vi "main_control_YJtoy.vi"() -> ()   [LabVIEW 2021]
uses:
  Addons/DAQ_Pulse_Gen/DAQ_Control_2.ctl
  Addons/DAQ_Pulse_Gen/DAQ_Control_1.ctl
  Ver_2/Config_File_Paths_v2.ctl
  Ver_2/ZI_Data_v2.ctl
  Addons/DAQ_Pulse_Gen/DAQ_Control_3 .ctl
  <vilib>/Utility/file.llb/Write Delimited Spreadsheet (DBL).vi
  <vilib>/gmath/NumericalOptimization/Nonlinear Curve Fit LM formula string.vi
  <vilib>/Utility/error.llb/Error Cluster From Error Code.vi
  <vilib>/ErrorRing/Error Ring.xnode
  <vilib>/Utility/Data Type/NI_Data Type.lvlib
  <vilib>/Analysis/NI_AALPro.lvlib
  <vilib>/gmath/NI_Gmath.lvlib
panel:
  out "Process name":string
  out "Initial_state_name":string
  out "tomography rotation memory (priv) 2":cluster{"Time":dbl[], dbl[]}[](array[cluster])
  out "MaxTime":dbl
  out "Process Array":cluster{"Timing 0":dbl[]}[](array[cluster])
  out "tomography rotation memory (priv)":cluster{"Time":dbl[], dbl[]}[](array[cluster])
  in  "pulses type (priv)":string[](array[string])=["None", "Y pi/2", "X pi/2"]
  in  "stop":bool
  in  "Tab Control":T1(tab)=enum."Design QPT"
  out "Config folder":string
  out "Chennel names\nare correct (?)":bool
  out "Channel map":map{string, i32}(c390)
  out "Pulses map [us]":map{string, dbl}(c390)
  out "Sampling data":T2={"Sample Numbers"=20000000, "Sample  Frequency (Hz)"=20000000}
  out "Resource Address":T3={"ZI Address"="DEV714", "VISA Keithley"="KEITHLEY"}
  in  "Period number":u32
  in  "Period [us]":dbl
  in  "Name of state (initial_state_)":string
  in  "Name of initial_state":u16(ring) items=["initial_state_01", "initial_state_02", "initial_state_03", "initial_state_04", "initial_state_05", "initial_state_06", "initial_state_07", "initial_state_08", "initial_state_09", "initial_state_10"]
  in  "Run tomography":bool
  in  "Run single FID":bool
  in  "Save for tomography":bool
  in  "Save single sequence":bool
  out "Pulses chart":cluster{dbl[], dbl[]}[](graph)
  in  "Reset sequence":bool
  in  "Channel":u16(ring) items=["LD pump", "LD repump", "LD probe", "pulse X", "pulse Y", "pulse Z", "Keithley ARM", "Keithley TRIG", "Accqusition TRIG", "Nonlinear coil", "None", "Tensor light shift", "pulse ZG"]
  in  "Add pulse advanced":bool
  in  "Physical channels":string[](array[string])
  in  "Add pulse":bool
  in  "Time [us]":dbl
  in  "Z pi/2":bool
  in  "Z pi":bool
  in  "Y pi/2":bool
  in  "Y pi":bool
  in  "X pi/2":bool
  in  "X pi":bool
  in  "Add pumping":bool
  in  "Pumping":T4(ring)
  in  "AOC":bool
  in  "X pi/4":bool
  in  "Save initial state":bool
  in  "Save  process":bool
  in  "Name of process (process_)":string
  in  "Name of process":u16(ring) items=["process_01", "process_02", "process_03", "process_04", "process_05", "process_06", "process_07", "process_08", "process_09", "process_10"]
  in  "Y pi/4":bool
  in  "Z pi/4":bool
  in  "Save multi Sequence":bool
  in  "Run QPT":bool
  in  "initial_state_show":u16(ring) items=["initial_state_01.ini", "initial_state_02.ini", "initial_state_03.ini", "initial_state_04.ini", "initial_state_05.ini", "initial_state_06.ini", "initial_state_07.ini", "initial_state_08.ini", "initial_state_09.ini"]
  in  "Choose init states":bool
  in  "State_update":bool
  out "State_List":string[](array[string]) caption="The Choosen States"
  in  "Delete init states":bool
  in  "Show init state":bool
  in  "Process_update":bool
  in  "Process_show":u16(ring) caption="initial_state_show" items=["process_01.ini", "process_02.ini", "process_03.ini", "process_04.ini", "process_05.ini", "process_06.ini", "process_07.ini", "process_08.ini", "process_09.ini", "process_10.ini"]
  in  "Choose the process":bool
  out "The Choosen Process":string
  out "Pulses chart 2":cluster{dbl[], dbl[]}[](graph)
  out "Pulses chart 3":cluster{dbl[], dbl[]}[](graph)
  in  "Save QPT":bool
  in  "Clear All states":bool
  in  "Multi-FID":bool
  in  "save":bool
  out "Rotation signal 3":cluster{"Time":dbl[], "Array":dbl[]}[](graph)
  out "w":dbl format="%#_3f"
  out "q":dbl format="%#_3f"
  out "g2":dbl format="%#_3f"
  out "g1":dbl format="%#_3f"
  out "C":dbl format="%#_3f"
  out "B":dbl format="%#_3f"
  out "A":dbl format="%#_3f"
  in  "Enum":T5(ring)
  in  "Fit model":bool
  out "Rotation signal":cluster{"Time":dbl[], dbl[]}(graph)
  out "Rotation spectrum":waveform(dbl)[](graph)
  out "Differential signal":cluster{"Time":dbl[], "X":dbl[]}[](graph)
  out "Intensity signal":cluster{"Time":dbl[], dbl[]}(graph)
  out "Polarimeter":dbl(knob) scale=-10.0..10.0
  in  "Run single FID 2":bool
  out "Progress":dbl(slide) scale=0.0..100.0
  in  "Number of repetition":u32=1 min=1 step=1
  in  "Signal in X or Y (?)":bool
  in  "Plot type":u16(ring) items=["None + [ None ]", "None + [ Y pi ]", "None + [ Z(pi/2)+Y(pi) ]", "Y pi/2 + [ None ]", "Y pi/2 + [ Y pi ]", "Y pi/2 + [ Z(pi/2)+Y(pi) ]", "X pi/2 + [ None ]", "X pi/2 + [ Y pi ]", "X pi/2 + [ Z(pi/2)+Y(pi) ]"]
  in  "Save raw data (?)":bool
  in  "Save CYCLOPS data (?)":bool
  out "Rotation signal":cluster{"Time":dbl[], dbl[]}(graph)
  in  "Run tomography 2":bool
  in  "Averaging":u8=1 min=1 step=1
  out "Differential signal":cluster{"Time":dbl[], "X":dbl[]}[](graph)
  out "Intensity signal":cluster{"Time":dbl[], dbl[]}(graph)
  out "Progress":dbl(slide) scale=0.0..100.0
  out "Rotation spectrum":waveform(dbl)[](graph)
  out "Rotation":cluster{"Time":dbl[], dbl[]}(graph)
  in  "Save raw data (?) 2":bool
  in  "Save CYCLOPS data (?) 2":bool
  out "Rotation spectrum 2":waveform(dbl)[](graph)
  out "Rotation signal 2":cluster{"Time":dbl[], dbl[]}(graph)
  out "Differential signal 2":cluster{"Time":dbl[], "X":dbl[]}[](graph)
  out "Intensity signal 2":cluster{"Time":dbl[], dbl[]}(graph)
  out "Single Tomography Progress":dbl(slide) scale=0.0..100.0
  out "Rotation 2":cluster{"Time":dbl[], dbl[]}(graph)
  in  "Averaging 2":u8=1 min=1 step=1
  in  "Run QPT 2":bool
  out "Current_QPT_order":i32
  out "QPT Progress":dbl(slide) scale=0.0..100.0
  # "To change that tab you need to go to block diagram"
  # "Probing will be added during saving"
  # "X"
  # "Y"
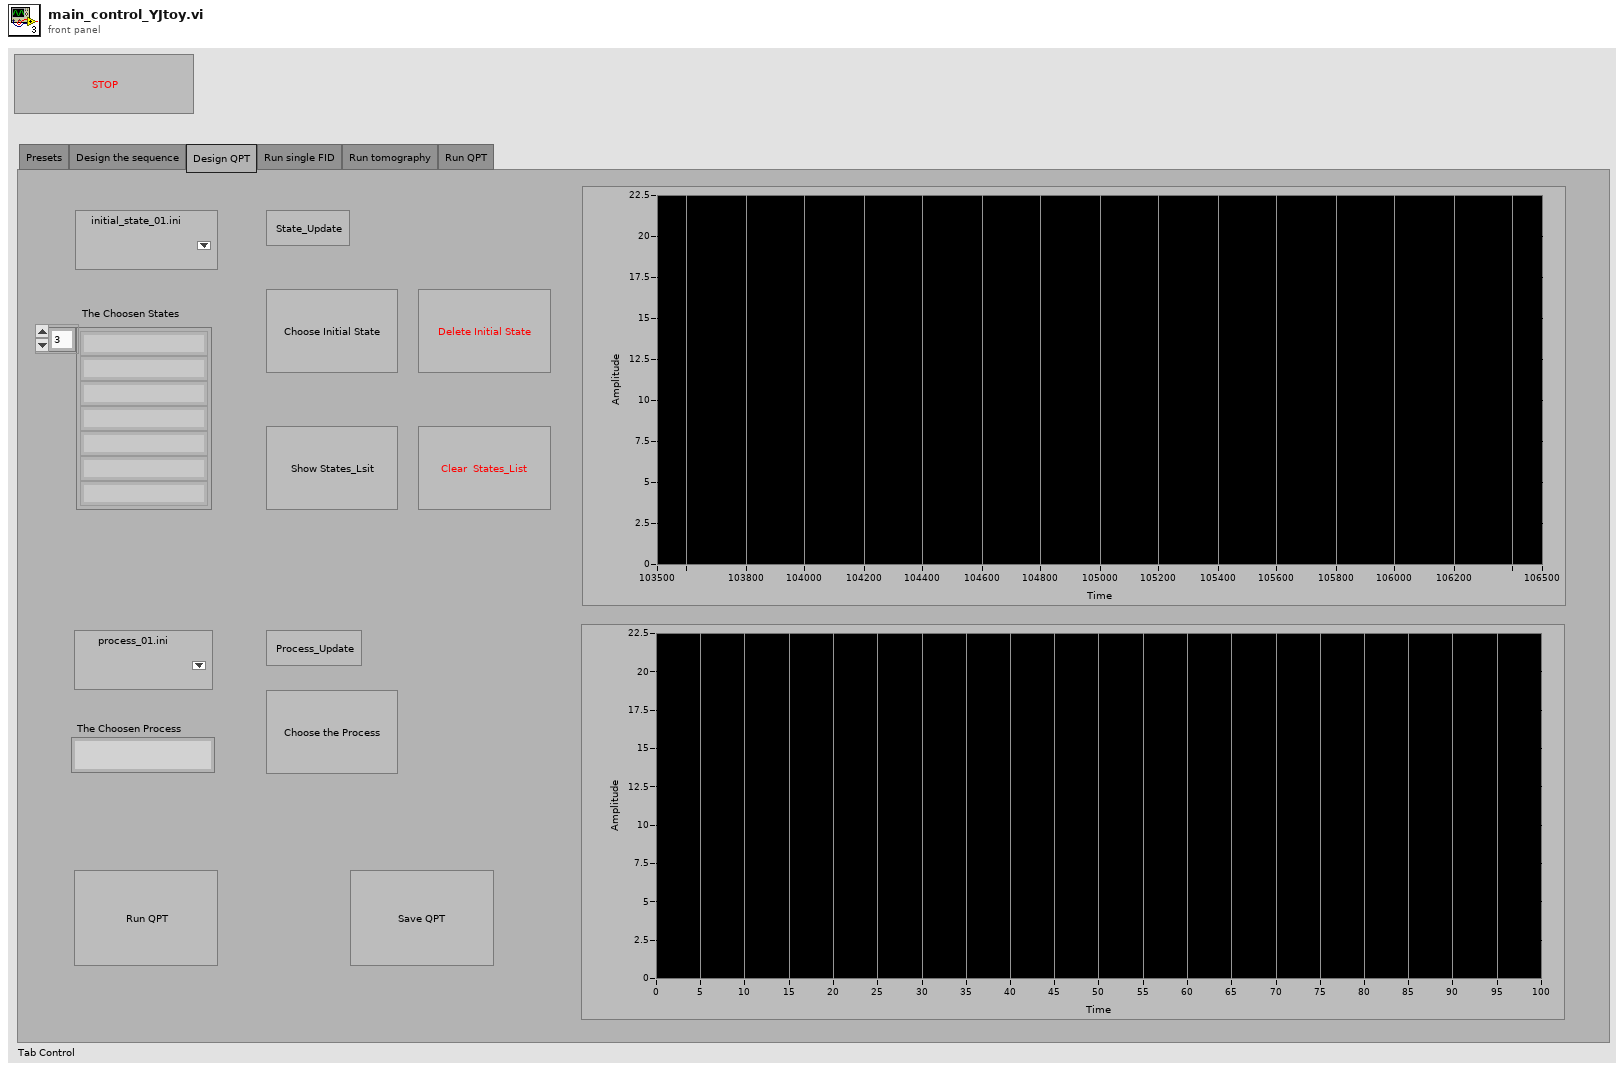
[diagram p1: front panel]
types:
  T1 = enum32{"Presets", "Design the sequence", "Design QPT", "Run single FID", "Run tomography", "Run QPT"}
  T2 = typedef "DAQ_Control_2.ctl" = cluster{"Sample Numbers":u32, "Sample  Frequency (Hz)":u32}
  T3 = cluster{"ZI Address":string, "VISA Keithley":refnum<visa-resource-name>}
  T4 = enum16{"Circular along X", "Linear in Y", "Linear in Z"}
  T5 = enum16{"Full", "A*Sin(w*t+q)*Exp(-g1*t)+C", "B*Exp(-q2*t)+C"}
  T6 = typedef "DAQ_Control_1.ctl" = cluster{"Port 2/line 6":cluster{"Timing 22":dbl[]}, "Port 2/line 5":cluster{"Timing 21":dbl[]}, "Port 2/line 4":cluster{"Timing 20":dbl[]}, "Port 2/line 3":cluster{"Timing 19":dbl[]}, "Port 2/line 2":cluster{"Timing 18":dbl[]}, "Port 2/line 1":cluster{"Timing 17":dbl[]}, "Port 2/line 0":cluster{"Timing 16":dbl[]}, "Port 1/line 7":cluster{"Timing 15":dbl[]}, "Port 1/line 6":cluster{"Timing 14":dbl[]}, "Port 1/line 5":cluster{"Timing 13":dbl[]}, "Port 1/line 4":cluster{"Timing 12":dbl[]}, "Port 1/line 3":cluster{"Timing 11":dbl[]}, "Port 1/line 2":cluster{"Timing 10":dbl[]}, "Port 1/line 1":cluster{"Timing 9":dbl[]}, "Port 1/line 0":cluster{"Timing 8":dbl[]}, "Port 0/line 7":cluster{"Timing 7\n":dbl[]}, "Port 0/line 6":cluster{"Timing 6\n":dbl[]}, "Port 0/line 5":cluster{"Timing 5\n":dbl[]}, "Port 0/line 4":cluster{"Timing 4\n":dbl[]}, "Port 0/line 3":cluster{"Timing 3\n":dbl[]}, "Port 0/line 2":cluster{"Timing 2":dbl[]}, "Port 0/line 1":cluster{"Timing 1\n":dbl[]}, "Port 0/line 0":cluster{"Timing 0":dbl[]}}
  T7 = typedef "Config_File_Paths_v2.ctl" = cluster{"ZI config file (.ini)":string, "Keithley config file (.ini)":string, "DAQ config file (.ini)":string}
  T8 = enum32{"Presets", "Design the sequence", "Design QPT", "Run single FID"}
  T9 = enum8{"Enabled", "Disabled", "Disabled and Grayed Out"}
  T10 = enum32{"Presets", "Design the sequence", "Design QPT", "Run single FID", "Run tomography"}
  T11 = cluster{"model":string, "Parameters":string[], "x":string}
  T12 = typedef "DAQ_Control_3 .ctl" = cluster{"Time Unit":enum16{"NanoSecond", "MicroSecond", "MilliSecond"}}
  T13 = typedef "ZI_Data_v2.ctl" = cluster{"R":dbl[], "Theta":dbl[], "X":dbl[], "Y":dbl[], "AuxIn0":dbl[], "AuxIn1":dbl[], "Frequency":dbl[], "DIO":dbl[], "Time":dbl[]}
  T14 = typedef "Resources_v2.ctl" = cluster{"ZI Handle":T15, "ZI ModHandle":T16, "VISA Keithley":refnum<visa-resource-name>}
  T15 = typedef "Zurich Instruments LabOne.lvlib/ziTypeHandle.ctl" = cluster{"handleValid":bool, "Conn":u64, "Path Prefix":string, "Handle":u64, "Connected":bool, "Clockbase(s)":dbl}
  T16 = typedef "Zurich Instruments LabOne.lvlib/ziTypeModHandle.ctl" = cluster{"handleValid":bool, "Conn":u64, "ModHandle":u64, "moduleID":string, "Path Prefix":string}
  T17 = typedef "Cutted_Data_v2.ctl" = cluster{"X":dbl[], "Y":dbl[], "Time":dbl[]}
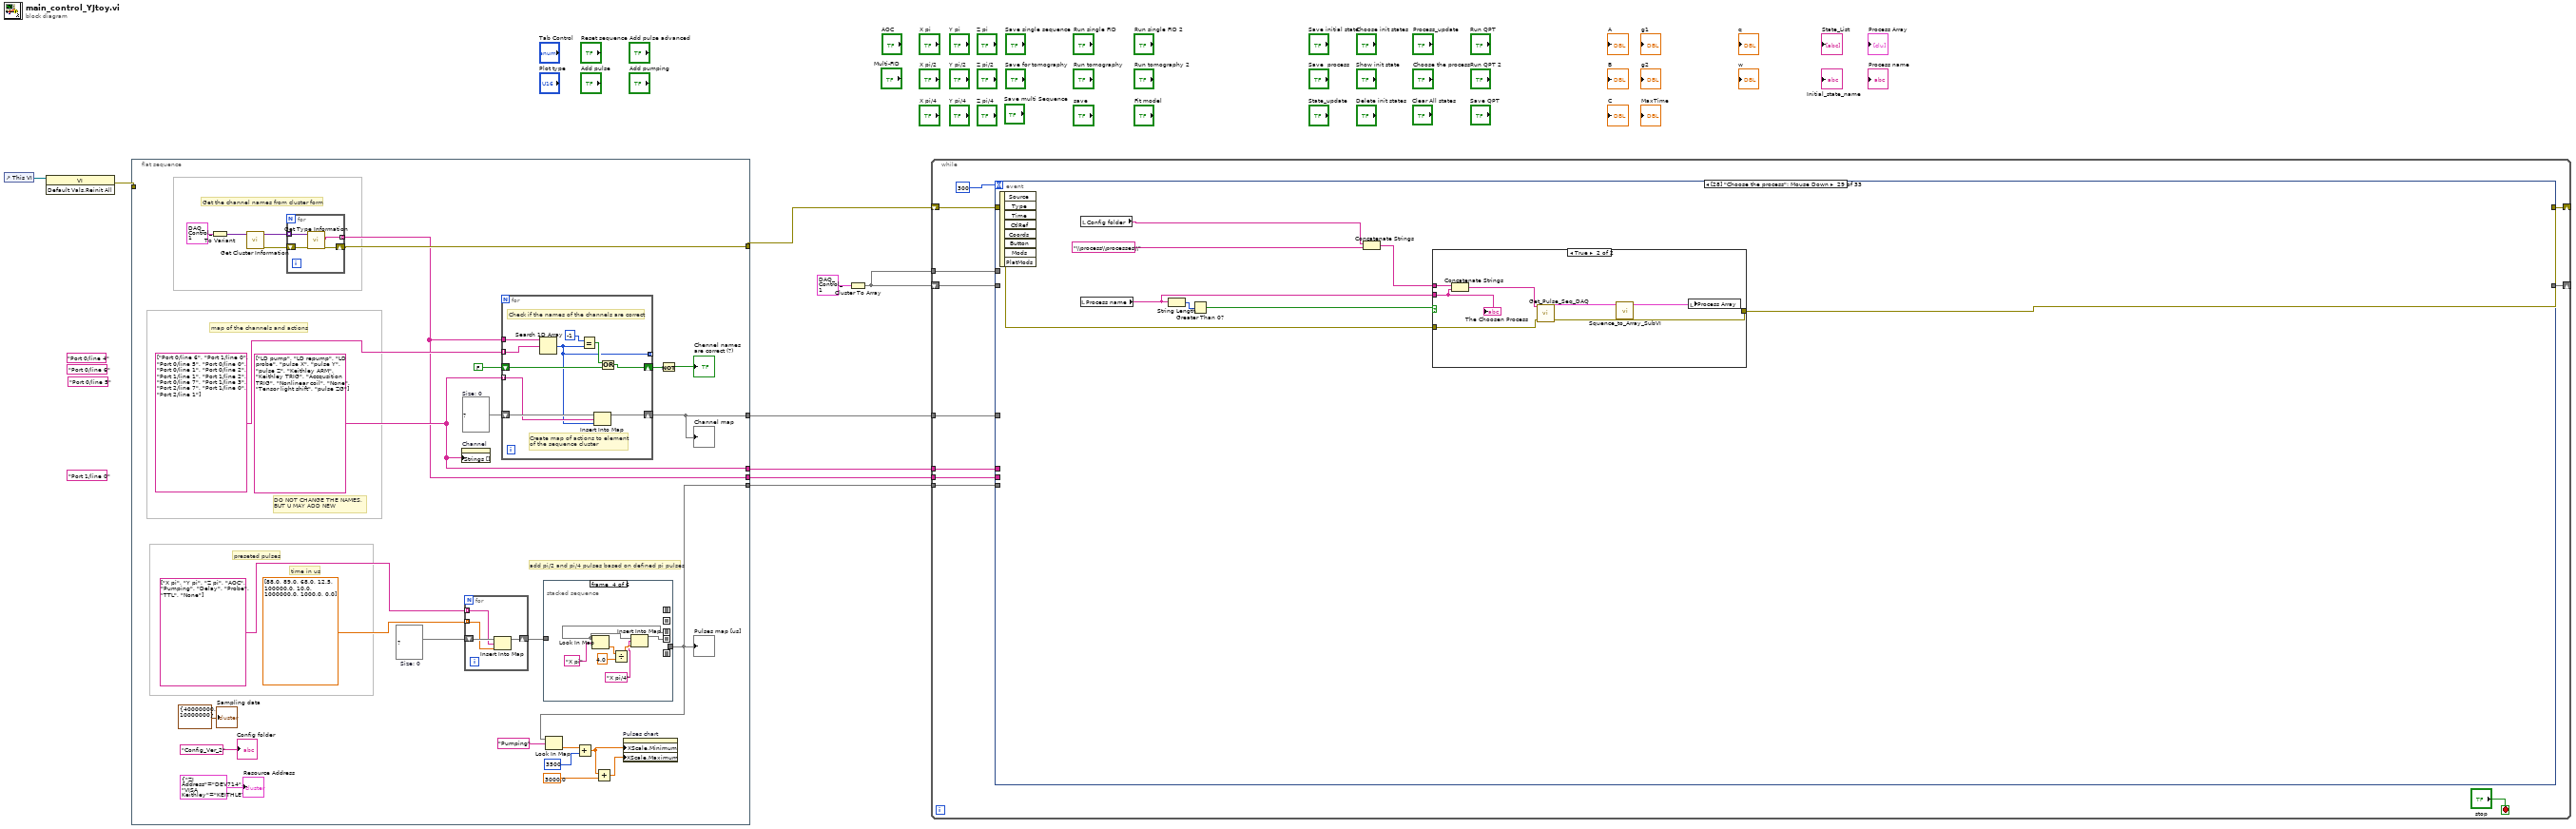
[diagram p0: block diagram]
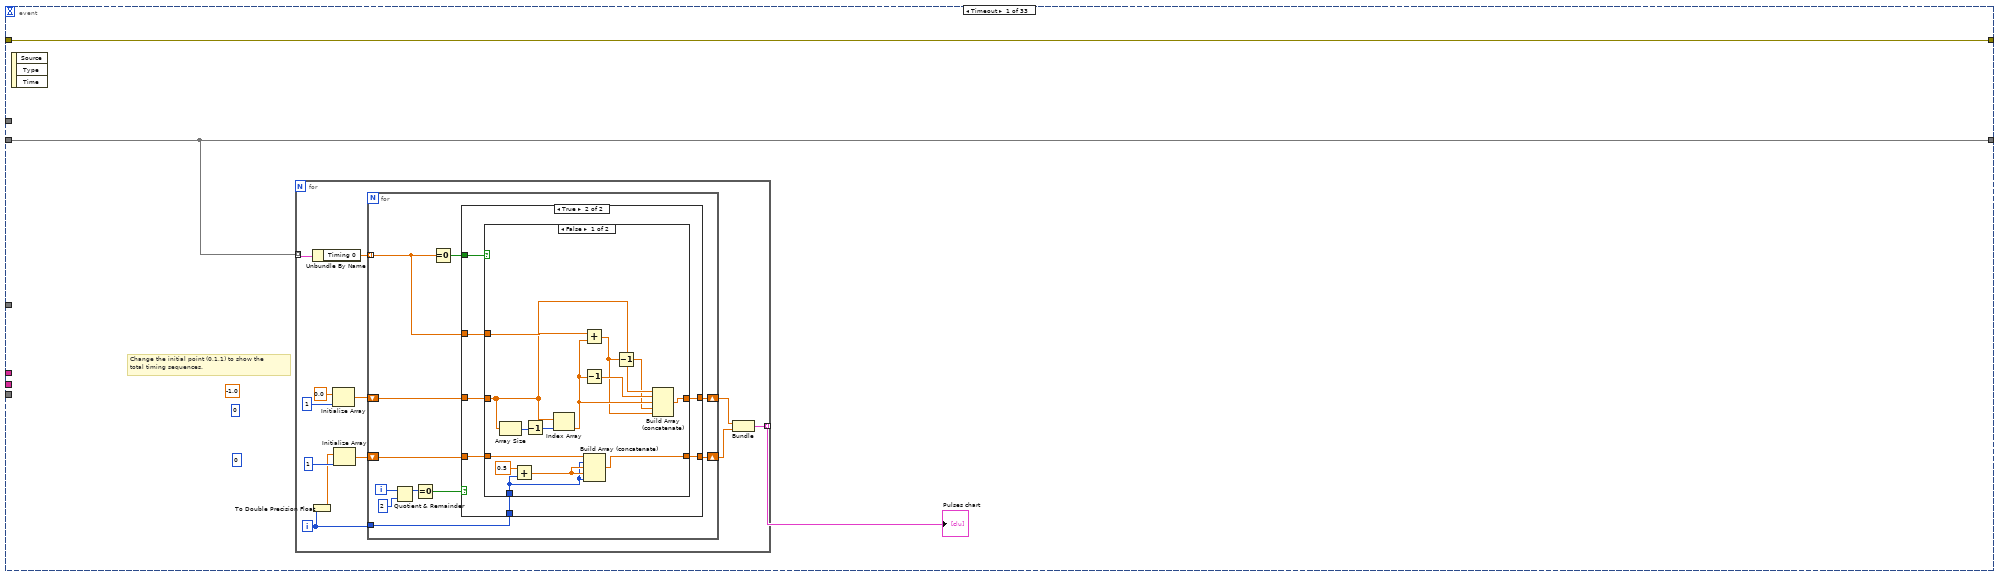
[diagram p2: hidden frame]
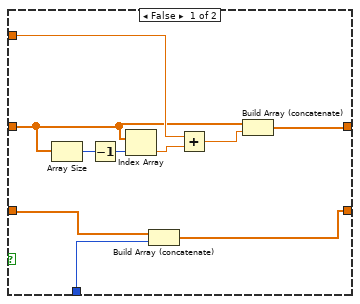
[diagram p3: hidden frame]
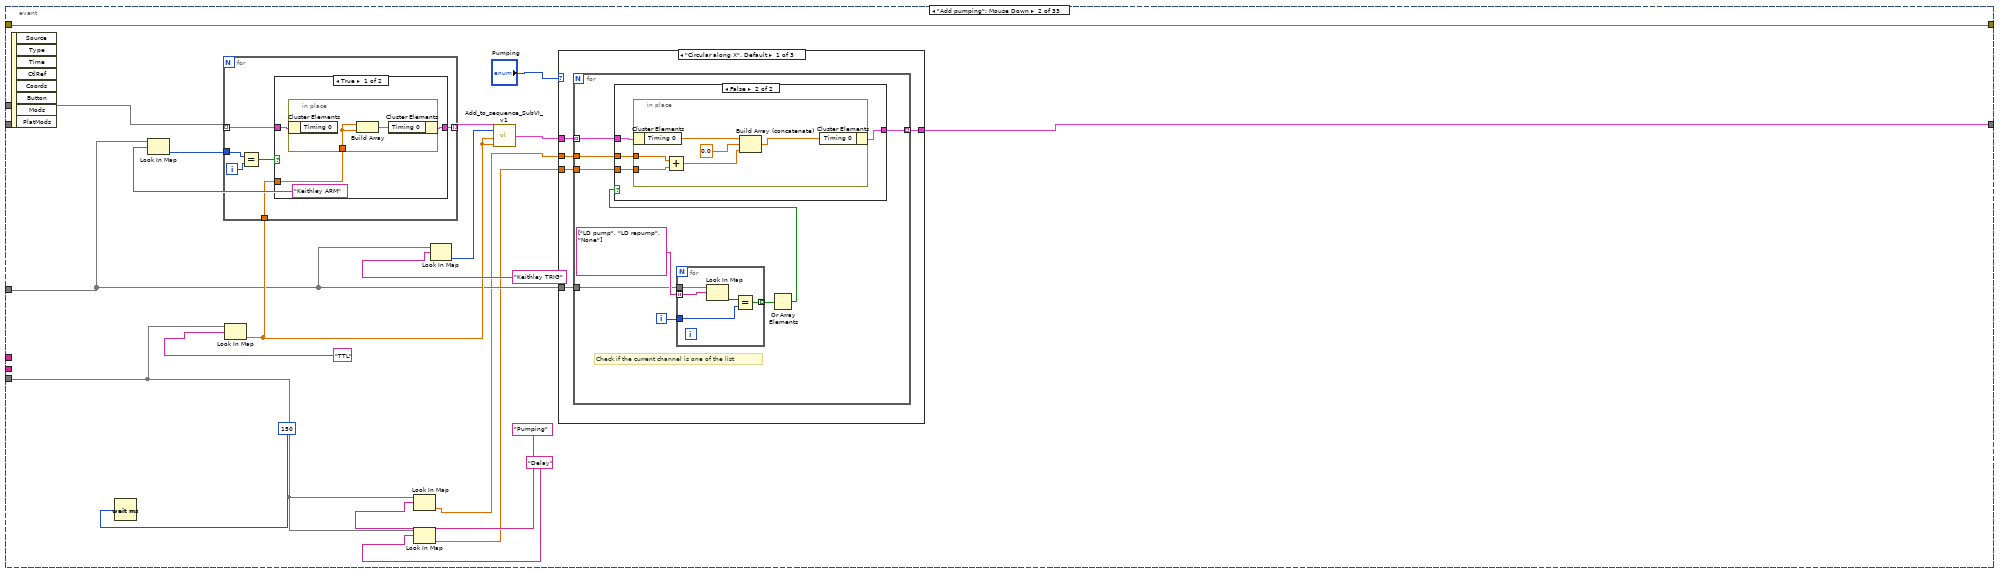
[diagram p5: hidden frame]
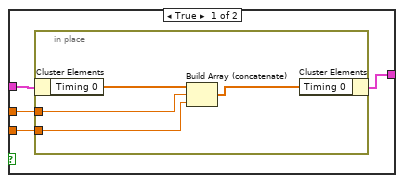
[diagram p6: hidden frame]
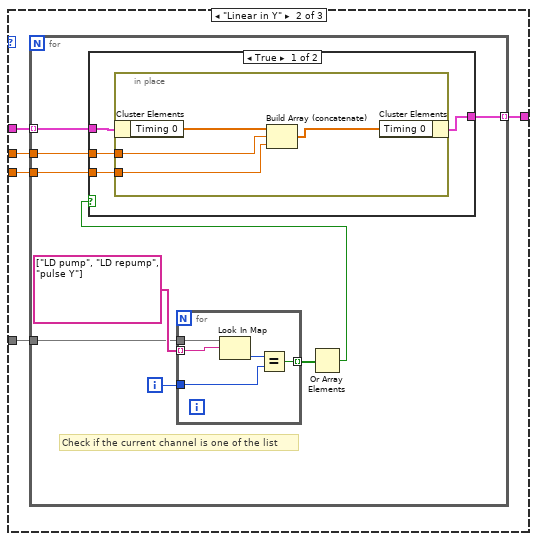
[diagram p7: hidden frame]
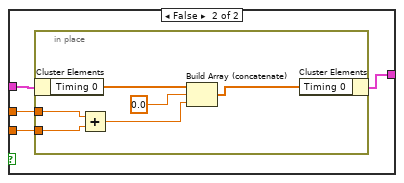
[diagram p8: hidden frame]
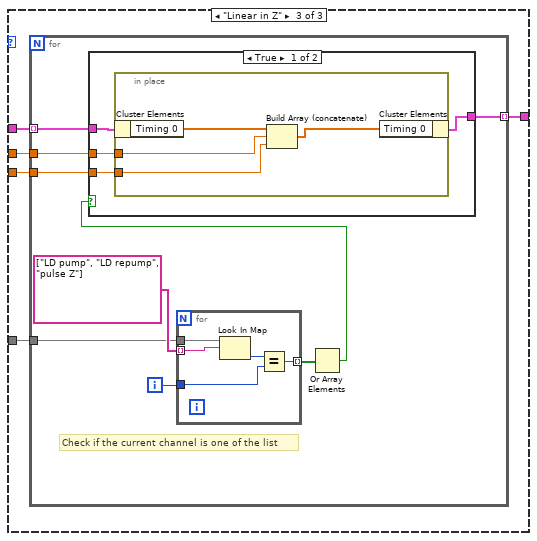
[diagram p9: hidden frame]
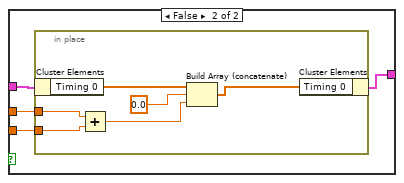
[diagram p10: hidden frame]
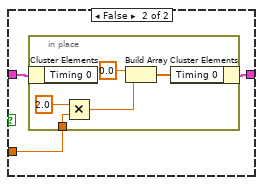
[diagram p11: hidden frame]
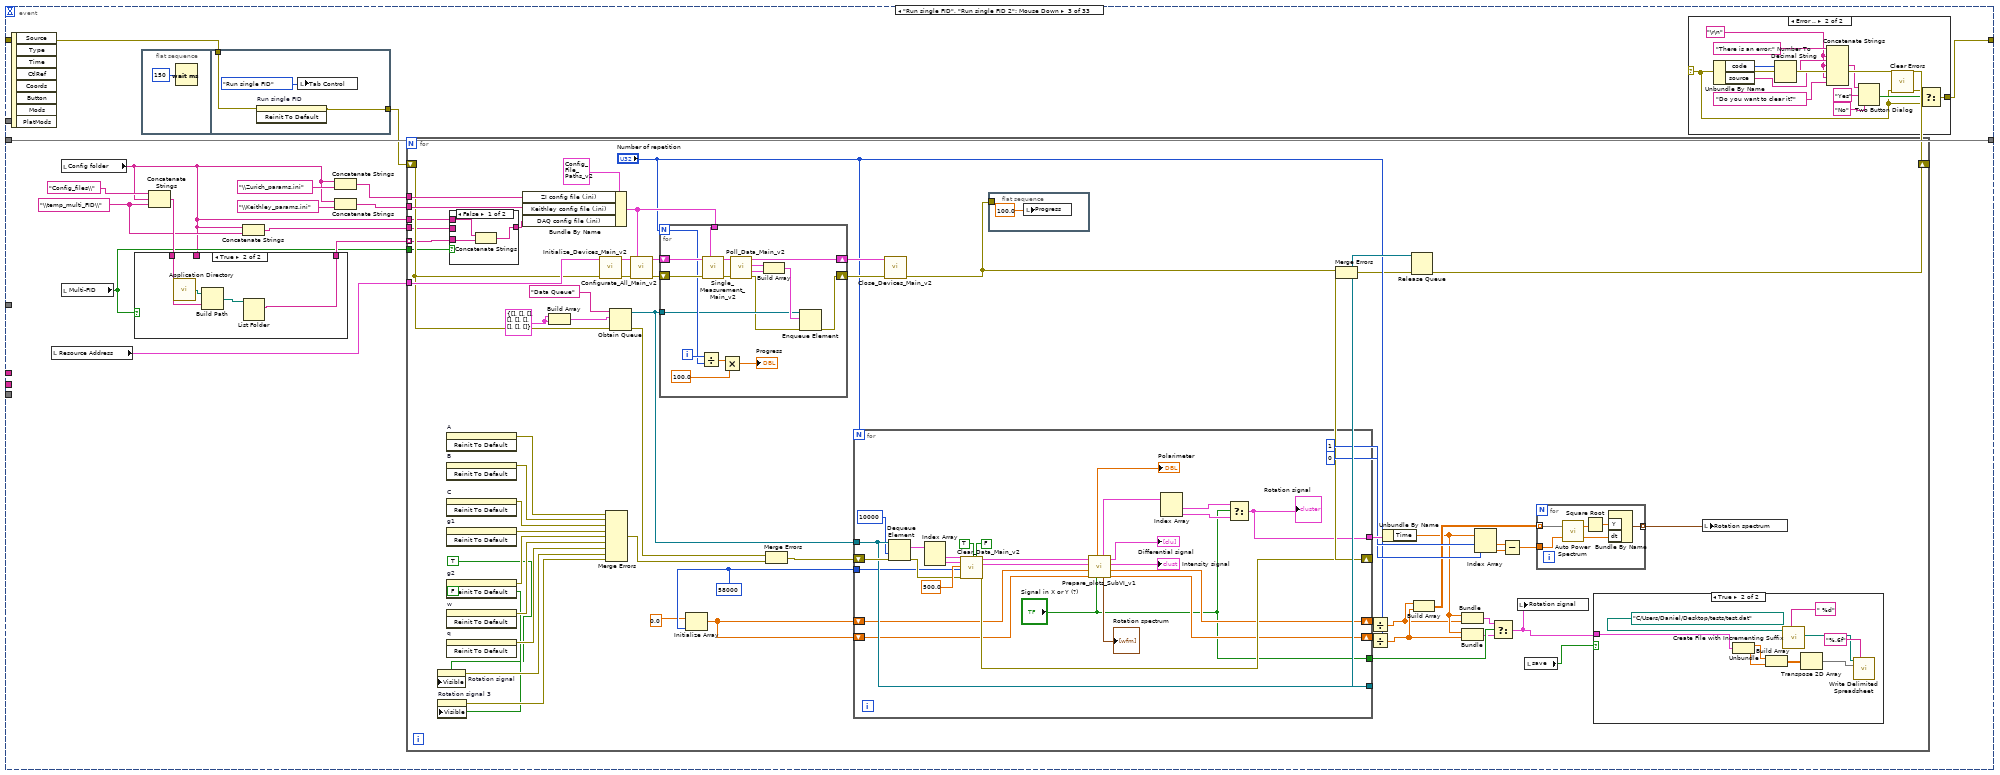
[diagram p12: hidden frame]
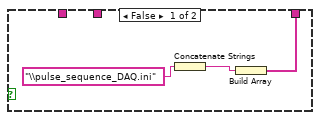
[diagram p13: hidden frame]
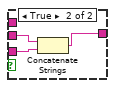
[diagram p14: hidden frame]
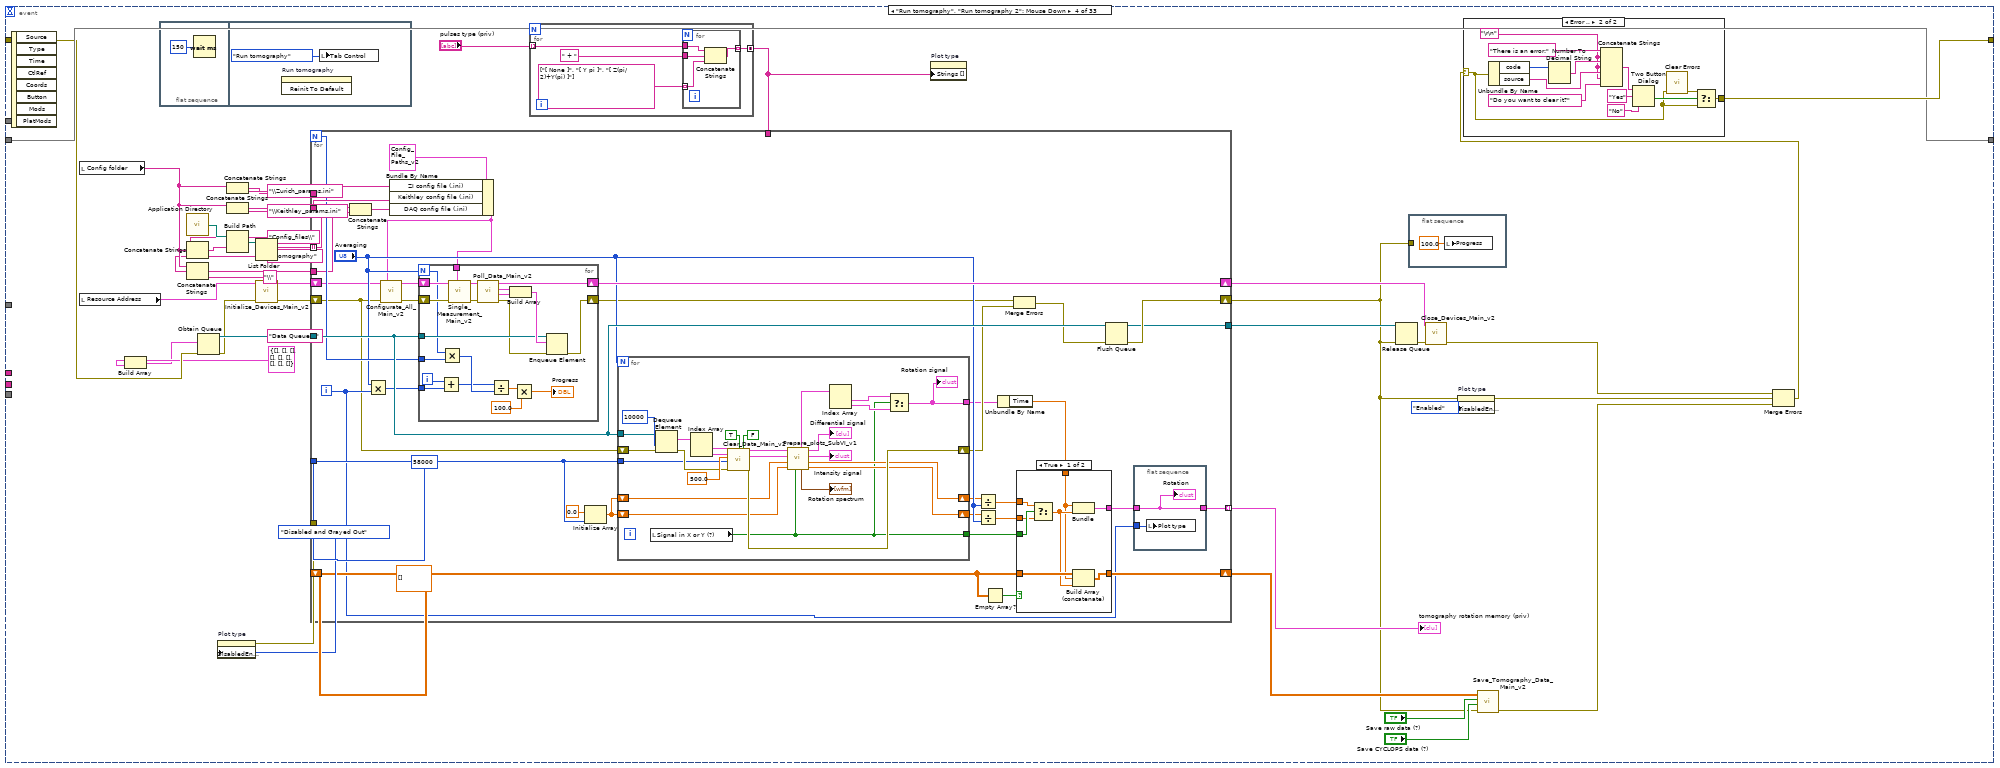
[diagram p17: hidden frame]
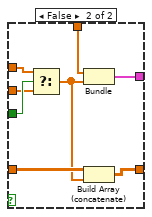
[diagram p18: hidden frame]
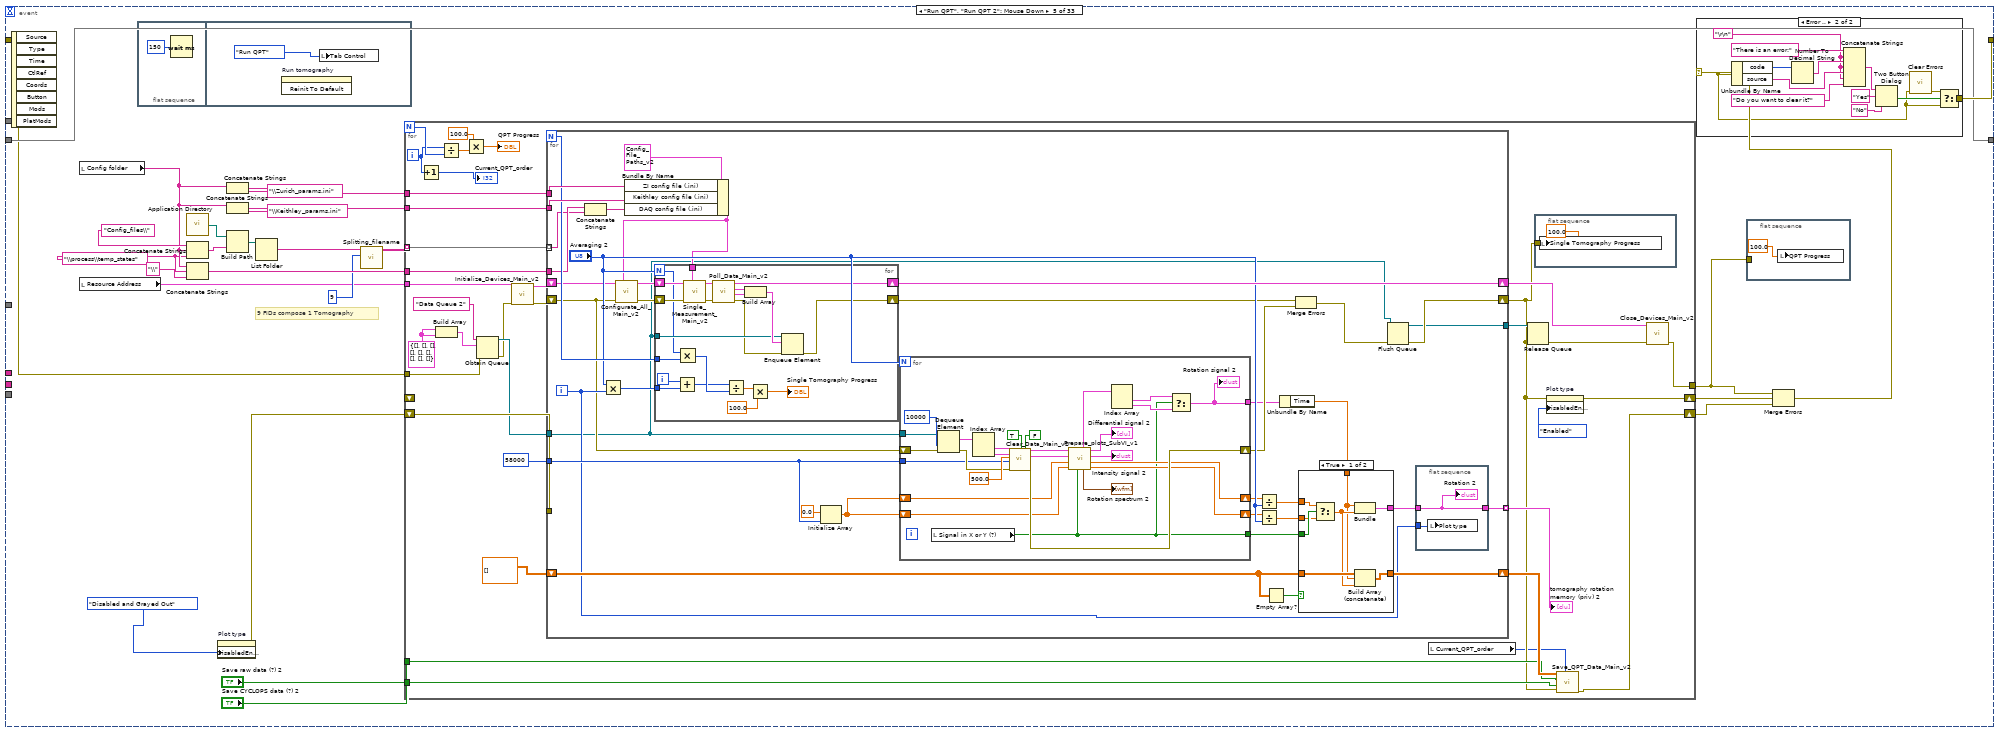
[diagram p20: hidden frame]
diagram:
  (unwired) "Port 0/line 5"
  (unwired) "Port 0/line 4"
  (unwired) "Port 1/line 0"
  (unwired) "Port 0/line 6"
  n1 = control-ref of="This VI"() -> (w2:refnum<vi>)
  n2 = invoke class="VI" method="Default Vals.Reinit All"(reference=w2) -> (error out=w1:errorcluster)  [unwired: 2 in, 2 out]
  n3 = flat-sequence {
    tunnel: [w23] -> w8
    tunnel: [w17] -> w7
    tunnel: [w22] -> w6
    tunnel: [w21] -> w5
    tunnel: [w20] -> w4
    tunnel: w1 -> [_]
    frame #0 {
      w27 = map{string, dbl} {}  # Size: 0
      w29 = map{string, i32} {}  # Size: 0
      w21 = string[] ["LD pump", "LD repump", "LD probe", "pulse X", "pulse Y", "pulse Z", "Keithley ARM", "Keithley TRIG", "Accqusition TRIG", "Nonlinear coil", "None", "Tensor light shift", "pulse ZG"]
      # "DO NOT CHANGE THE NAMES,\nBUT U MAY ADD NEW"
      # "add pi/2 and pi/4 pulses based on defined pi pulses"
      # "preseted pulses"
      # "time in us"
      # "map of the channels and actions"
      # "Get the channel names from cluster form"
      n4 = To Variant(anything=T6 {"Port 2/line 6"={"Timing 22"=[]}, "Port 2/line 5"={"Timing 21"=[]}, "Port 2/line 4"={"Timing 20"=[]}, "Port 2/line 3"={"Timing 19"=[]}, "Port 2/line 2"={"Timing 18"=[]}, "Port 2/line 1"={"Timing 17"=[]}, "Port 2/line 0"={"Timing 16"=[]}, "Port 1/line 7"={"Timing 15"=[]}, "Port 1/line 6"={"Timing 14"=[]}, "Port 1/line 5"={"Timing 13"=[]}, "Port 1/line 4"={"Timing 12"=[]}, "Port 1/line 3"={"Timing 11"=[]}, "Port 1/line 2"={"Timing 10"=[]}, "Port 1/line 1"={"Timing 9"=[]}, "Port 1/line 0"={"Timing 8"=[]}, "Port 0/line 7"={"Timing 7\n"=[]}, "Port 0/line 6"={"Timing 6\n"=[]}, "Port 0/line 5"={"Timing 5\n"=[]}, "Port 0/line 4"={"Timing 4\n"=[]}, "Port 0/line 3"={"Timing 3\n"=[]}, "Port 0/line 2"={"Timing 2"=[]}, "Port 0/line 1"={"Timing 1\n"=[]}, "Port 0/line 0"={"Timing 0"=[]}} ("Sequence")) -> (Variant=w35:variant)
      n5 = call <vilib>:"Get Cluster Information.vi"("variant"=w35) -> ("error out"=w34:errorcluster, "cluster elements"=w33:variant[])  [unwired: 9 in]
      n6 = for {
        tunnel: w33 -> [w96] mode=indexing
        shift-right: [w94] -> w22
        shift-left: w34 -> [w95]
        tunnel: [w93] -> w20 mode=indexing
        n7 = call <vilib>:"Get Type Information.vi"("error in (no error)"=w95, "variant"=w96) -> ("error out"=w94:errorcluster, "name"=w93:string)  [unwired: 5 in, 3 out]
      }
      n8 = property on="Channel" class="Ring (strict)"("Strings []"=w21) -> ()  [unwired: 2 in, 2 out]
      n9 = for {
        shift-right: [w79] -> w24
        shift-left: w27 -> [w82]
        tunnel: string[] ["X pi", "Y pi", "Z pi", "AOC", "Pumping", "Delay", "Probe", "TTL", "None"] -> [w81] mode=indexing
        tunnel: dbl[] [88.0, 89.0, 68.0, 12.5, 100000.0, 10.0, 1000000.0, 1000.0, 0.0] -> [w80] mode=indexing
        n10 = Insert Into Map(map in=w82, key=w81, value=w80) -> (map out=w79:map{string, dbl})  [unwired: 2 out]
      }
      n11 = for {
        tunnel: w20 -> [w92]
        tunnel: string[] ["Port 0/line 6", "Port 1/line 0", "Port 0/line 5", "Port 0/line 0", "Port 0/line 1", "Port 0/line 2", "Port 1/line 1", "Port 1/line 2", "Port 0/line 7", "Port 1/line 3", "Port 2/line 7", "Port 1/line 0", "Port 2/line 1"] -> [w83] mode=indexing
        shift-right: [w88] -> w31
        shift-left: FALSE -> [w89]
        tunnel: [w85] -> _ mode=indexing
        shift-right: [w84] -> w23
        shift-left: w29 -> [w87]
        tunnel: w21 -> [w86] mode=indexing
        # "Create map of actions to element\nof the sequence cluster"
        # "Check if the names of the channels are correct"
        n12 = Search 1D Array(1D array=w92, element=w83) -> (index of element=w85:i32)  [unwired: 1 in]
        n13 = Equal?(x=-1, y=w85) -> (x = y?=w90:bool)
        n14 = Insert Into Map(map in=w87, key=w86, value=w85) -> (map out=w84:map{string, i32})  [unwired: 2 out]
        n15 = Or(x=w90, y=w89) -> (x .or. y?=w88:bool)
      }
      "Channel map" <- w23
      n16 = stacked-sequence {
        seq-local: [w37 _ _ _ _ _] -> [_ w44 _ _ _ _]
        seq-local: [_ w45 _ _ _ _] -> [_ _ w52 _ _ _]
        seq-local: [_ _ w51 _ _ _] -> [_ _ _ w63 _ _]
        seq-local: [_ _ _ w59 _ _] -> [_ _ _ _ w71 _]
        seq-local: [_ _ _ _ w70 _] -> [_ _ _ _ _ w78]
        tunnel: w24 -> [w41 _ _ _ _ _]
        tunnel: [_ _ _ _ _ w77] -> w17
        frame #0 {
          n17 = Look In Map(map=w41, key="X pi") -> (value=w39:dbl)  [unwired: 1 in, 1 out]
          n18 = Divide(x=w39, y=2.0) -> (x/y=w40:dbl)
          n19 = Insert Into Map(map in=w41, key="X pi/2", value=w40) -> (map out=w37:map{string, dbl})  [unwired: 2 out]
        }
        frame #1 {
          n20 = Look In Map(map=w44, key="Y pi") -> (value=w50:dbl)  [unwired: 1 in, 1 out]
          n21 = Divide(x=w50, y=2.0) -> (x/y=w49:dbl)
          n22 = Insert Into Map(map in=w44, key="Y pi/2", value=w49) -> (map out=w45:map{string, dbl})  [unwired: 2 out]
        }
        frame #2 {
          n23 = Look In Map(map=w52, key="Z pi") -> (value=w54:dbl)  [unwired: 1 in, 1 out]
          n24 = Divide(x=w54, y=2.0) -> (x/y=w55:dbl)
          n25 = Insert Into Map(map in=w52, key="Z pi/2", value=w55) -> (map out=w51:map{string, dbl})  [unwired: 2 out]
        }
        frame #3 {
          n26 = Look In Map(map=w63, key="X pi") -> (value=w62:dbl)  [unwired: 1 in, 1 out]
          n27 = Divide(x=w62, y=4.0) -> (x/y=w60:dbl)
          n28 = Insert Into Map(map in=w63, key="X pi/4", value=w60) -> (map out=w59:map{string, dbl})  [unwired: 2 out]
        }
        frame #4 {
          n29 = Look In Map(map=w71, key="Y pi") -> (value=w68:dbl)  [unwired: 1 in, 1 out]
          n30 = Divide(x=w68, y=4.0) -> (x/y=w66:dbl)
          n31 = Insert Into Map(map in=w71, key="Y pi/4", value=w66) -> (map out=w70:map{string, dbl})  [unwired: 2 out]
        }
        frame #5 {
          n32 = Look In Map(map=w78, key="Z pi") -> (value=w75:dbl)  [unwired: 1 in, 1 out]
          n33 = Divide(x=w75, y=4.0) -> (x/y=w73:dbl)
          n34 = Insert Into Map(map in=w78, key="Z pi/4", value=w73) -> (map out=w77:map{string, dbl})  [unwired: 2 out]
        }
      }
      "Pulses map [us]" <- w17
      n35 = Look In Map(map=w17, key="Pumping") -> (value=w19:dbl)  [unwired: 1 in, 1 out]
      n36 = Add(x=w19, y=3500) -> (x+y=w16:dbl)
      n37 = Add(x=w16, y=3000.0) -> (x+y=w14:dbl)
      n38 = property on="Pulses chart" class="XYGraph (strict)"("XScale.Minimum"=w16, "XScale.Maximum"=w14) -> ()  [unwired: 2 in, 2 out]
      n39 = Not(x=w31) -> (.not. x?=→"Chennel names\nare correct (?)":bool)
      "Sampling data" <- T2 {"Sample Numbers"=40000000, "Sample  Frequency (Hz)"=10000000} ("Sampling data")
      "Config folder" <- "Config_Ver_2" ("Filename (ini)")
      "Resource Address" <- T3 {"ZI Address"="DEV714", "VISA Keithley"="KEITHLEY"} ("Resource Address")
    }
  }
  n40 = Cluster To Array(cluster=T6 {"Port 2/line 6"={"Timing 22"=[]}, "Port 2/line 5"={"Timing 21"=[]}, "Port 2/line 4"={"Timing 20"=[]}, "Port 2/line 3"={"Timing 19"=[]}, "Port 2/line 2"={"Timing 18"=[]}, "Port 2/line 1"={"Timing 17"=[]}, "Port 2/line 0"={"Timing 16"=[]}, "Port 1/line 7"={"Timing 15"=[]}, "Port 1/line 6"={"Timing 14"=[]}, "Port 1/line 5"={"Timing 13"=[]}, "Port 1/line 4"={"Timing 12"=[]}, "Port 1/line 3"={"Timing 11"=[]}, "Port 1/line 2"={"Timing 10"=[]}, "Port 1/line 1"={"Timing 9"=[]}, "Port 1/line 0"={"Timing 8"=[]}, "Port 0/line 7"={"Timing 7\n"=[]}, "Port 0/line 6"={"Timing 6\n"=[]}, "Port 0/line 5"={"Timing 5\n"=[]}, "Port 0/line 4"={"Timing 4\n"=[]}, "Port 0/line 3"={"Timing 3\n"=[]}, "Port 0/line 2"={"Timing 2"=[]}, "Port 0/line 1"={"Timing 1\n"=[]}, "Port 0/line 0"={"Timing 0"=[]}} ("Sequence")) -> (array=w3:cluster{"Timing 0":dbl[]}[])
  n41 = while {
    shift-right: [w98] -> _
    shift-left: w3 -> [w107]
    tunnel: w8 -> [w106]
    tunnel: w7 -> [w97]
    shift-right: [w102] -> _
    shift-left: w6 -> [w103]
    tunnel: w5 -> [w101]
    tunnel: w4 -> [w100]
    tunnel: w3 -> [w99]
    stop <- "stop" stop-if-true
    n42 = event shown="[28] \"Choose the process\": Mouse Down" {
      selector: _ -> [_ _ _ _ _ _ _ _ _ _ _ _ _ _ _ _ _ _ _ _ _ _ _ _ _ _ _ _ _ _ _ _ _]
      dyn-events: _ -> [_ _ _ _ _ _ _ _ _ _ _ _ _ _ _ _ _ _ _ _ _ _ _ _ _ _ _ _ _ _ _ _ _]
      timeout: 300 -> [_ _ _ _ _ _ _ _ _ _ _ _ _ _ _ _ _ _ _ _ _ _ _ _ _ _ _ _ _ _ _ _ _]
      tunnel: w107 -> [w110 _ w327 w520 w675 w838 _ w1001 w1006 w1018 w1029 w1041 w1053 w1065 w1077 w1089 w1101 w1117 w1146 w1185 w1266 w1387 w1529 w1576 _ _ _ _ _ _ _ _ _]
      tunnel: w106 -> [_ w172 _ _ _ _ _ w985 w1013 w1025 w1036 w1048 w1060 w1072 w1084 w1096 w1108 w1122 _ w1198 w1268 w1392 _ _ w1640 _ _ _ _ _ _ _ _]
      tunnel: w97 -> [_ w171 _ _ _ _ _ w983 w1007 w1019 w1034 w1042 w1054 w1066 w1078 w1090 w1102 w1118 w1138 w1195 w1267 w1391 _ _ w1639 _ _ _ _ _ _ _ _]
      tunnel: [w110 w169 w327 w520 w675 w838 _ w978 w1005 w1017 w1028 w1040 w1052 w1064 w1076 w1088 w1100 w1116 w1135 w1185 _ w1387 w1529 w1576 _ _ _ _ _ _ _ _ w2013] -> w98
      tunnel: w103 -> [w109 w185 w326 w514 w657 w839 w881 w989 w1009 w1021 _ w1044 w1056 w1068 w1080 w1092 w1104 w1120 w1142 w1180 w1256 w1385 w1530 w1577 w1626 w1737 w1832 w1930 w1949 w1961 w1982 w2010 w2014]
      tunnel: [w109 w185 w324 w524 w678 w839 _ w989 w1009 w1021 _ w1044 w1056 w1068 w1080 w1092 w1104 w1120 w1142 w1179 w1263 w1384 w1531 w1578 w1647 w1736 w1825 w1925 w1943 w1968 w1979 w2009 w2014] -> w102
      tunnel: w101 -> [_ _ _ _ _ _ _ _ _ _ _ _ _ _ _ _ _ w1113 _ _ _ _ _ _ _ _ _ _ _ _ _ _ _]
      tunnel: w100 -> [_ _ _ _ _ _ _ _ _ _ _ _ _ _ _ _ _ _ w1144 _ _ _ _ _ _ _ _ _ _ _ _ _ _]
      tunnel: w99 -> [_ w168 _ _ _ _ _ _ _ _ _ _ _ _ _ _ _ _ _ _ _ _ _ _ _ _ _ _ _ _ _ _ w2013]
      event Timeout {
        (unwired) 0 ("dimension size")
        (unwired) 0 ("dimension size")
        (unwired) -1.0 ("element")
        # "Change the initial point (0,1,1) to show the \ntotal timing sequences."
        n43 = event-data() -> ()  [unwired: 1 in, 3 out]
        n44 = for {
          tunnel: w110 -> [w122] mode=indexing
          tunnel: [w111] -> w108 mode=indexing
          i -> [w114]
          n45 = To Double Precision Float(number=w114) -> (double precision float=w118:dbl)
          n46 = Unbundle By Name(w122) -> ("Timing 0"=w121:dbl[])
          n47 = Initialize Array(0.0 ("element"), 1 ("dimension size")) -> (w115:dbl[])
          n48 = Initialize Array(w118, 1 ("dimension size")) -> (w119:dbl[])
          n49 = for {
            tunnel: w121 -> [w124] mode=indexing
            shift-right: [w126] -> w112
            shift-left: w119 -> [w125]
            shift-right: [w128] -> w113
            shift-left: w115 -> [w127]
            tunnel: w114 -> [w123]
            i -> [w133]
            n50 = Quotient & Remainder(x=w133, y=2) -> (x-y*floor(x/y)=w131:i32)  [unwired: 1 out]
            n51 = Equal To 0?(x=w131) -> (x = 0?=w130:bool)
            n52 = Equal To 0?(x=w124) -> (x = 0?=w129:bool)
            n53 = case shown="True" w130 {
              tunnel: w129 -> [_ w150]
              tunnel: [w134 w149] -> w128
              tunnel: w127 -> [w136 w148]
              tunnel: [w141 w147] -> w126
              tunnel: w125 -> [w142 w146]
              tunnel: w124 -> [w137 w145]
              tunnel: w123 -> [w143 w144]
              frame False {
                n54 = Array Size(array=w136) -> (size(s)=w140:i32)
                n55 = Decrement(x=w140) -> (x-1=w139:i32)
                n56 = Index Array(array=w136, index=w139) -> (element=w138:dbl)
                n57 = Build Array (concatenate)(w142, w143) -> (w141:dbl[])
                n58 = Add(x=w137, y=w138) -> (x+y=w135:dbl)
                n59 = Build Array (concatenate)(w136, w135) -> (w134:dbl[])
              }
              frame True {
                n60 = case shown="False" w150 {
                  tunnel: [w161 w166] -> w149
                  tunnel: w148 -> [w155 w166]
                  tunnel: [w157 w165] -> w147
                  tunnel: w146 -> [w164 w165]
                  tunnel: w145 -> [w162 _]
                  tunnel: w144 -> [w158 _]
                  frame False {
                    n61 = Array Size(array=w155) -> (size(s)=w163:i32)
                    n62 = Add(x=0.5, y=w158) -> (x+y=w159:dbl)
                    n63 = Decrement(x=w163) -> (x-1=w156:i32)
                    n64 = Index Array(array=w155, index=w156) -> (element=w153:dbl)
                    n65 = Add(x=w162, y=w153) -> (x+y=w152:dbl)
                    n66 = Decrement(x=w153) -> (x-1=w154:dbl)
                    n67 = Build Array (concatenate)(w164, w158, w159, w159, w158) -> (w157:dbl[])
                    n68 = Decrement(x=w152) -> (x-1=w151:dbl)
                    n69 = Build Array (concatenate)(w155, w154, w153, w151, w152) -> (w161:dbl[])
                  }
                  frame True {
                  }
                }
              }
            }
          }
          n70 = Bundle(w113, w112) -> (w111:cluster{dbl[], dbl[]})  [unwired: 1 in]
        }
        "Pulses chart" <- w108
      }
      event "Add pumping": Mouse Down {
        n71 = event-data() -> ()  [unwired: 1 in, 8 out]
        n72 = Wait (ms)(milliseconds to wait=u32 150) -> ()  [unwired: 1 out]
        n73 = Look In Map(map=w172, key="Keithley ARM") -> (value=w182:i32)  [unwired: 1 in, 1 out]
        n74 = Look In Map(map=w171, key="TTL") -> (value=w177:dbl)  [unwired: 1 in, 1 out]
        n75 = for {
          tunnel: w168 -> [w299] mode=indexing
          tunnel: w182 -> [w301]
          tunnel: w177 -> [w298]
          tunnel: [w297] -> w180 mode=indexing
          i -> [w302]
          n76 = Equal?(x=w301, y=w302) -> (x = y?=w300:bool)
          n77 = case shown="True" w300 {
            tunnel: w299 -> [w305 w310]
            tunnel: w298 -> [w304 w309]
            tunnel: [w303 w308] -> w297
            frame True {
              n78 = in-place {
                in-place-border: w304 -> [w307]
                n79 = in-place-cluster #1(w305) -> ()  [unwired: 1 out]
                n80 = Build Array(w307, w307) -> (w306:dbl[])
                n81 = in-place-cluster #1("Timing 0"=w306) -> (w303:cluster{"Timing 0":dbl[]})
              }
            }
            frame False {
              n82 = in-place {
                in-place-border: w309 -> [w313]
                n83 = in-place-cluster #2(w310) -> ()  [unwired: 1 out]
                n84 = Multiply(x=2.0, y=w313) -> (x*y=w311:dbl)
                n85 = Build Array(0.0 ("element"), w311) -> (w315:dbl[])
                n86 = in-place-cluster #2("Timing 0"=w315) -> (w308:cluster{"Timing 0":dbl[]})
              }
            }
          }
        }
        n87 = Look In Map(map=w171, key="Pumping") -> (value=w167:dbl)  [unwired: 1 in, 1 out]
        n88 = Look In Map(map=w171, key="Delay") -> (value=w170:dbl)  [unwired: 1 in, 1 out]
        n89 = Look In Map(map=w172, key="Keithley TRIG") -> (value=w178:i32)  [unwired: 1 in, 1 out]
        n90 = call "Add_to_sequence_SubVI_v1.vi"("Delay [us]"=w177, "Pulse length [us]"=w177, "Channel number"=w178, "Array sequence in"=w180) -> ("Array sequence out"=w175:cluster{"Timing 0":dbl[]}[])
        n91 = case shown="\"Circular along X\", Default" "Pumping" {
          tunnel: w175 -> [w190 w227 w264]
          tunnel: w172 -> [w189 w226 w263]
          tunnel: w167 -> [w188 w225 w262]
          tunnel: w170 -> [w187 w224 w261]
          tunnel: [w186 w223 w260] -> w169
          frame "Circular along X", Default {
            n92 = for {
              tunnel: w190 -> [w194] mode=indexing
              tunnel: w189 -> [w196]
              tunnel: w188 -> [w193]
              tunnel: w187 -> [w192]
              tunnel: [w191] -> w186 mode=indexing
              i -> [w197]
              # "Check if the current channel is one of the list"
              n93 = for {
                tunnel: w196 -> [w221]
                tunnel: w197 -> [w220]
                tunnel: [w219] -> w199 mode=indexing
                tunnel: string[] ["LD pump", "LD repump", "None"] -> [w218] mode=indexing
                n94 = Look In Map(map=w221, key=w218) -> (value=w222:i32)  [unwired: 1 in, 1 out]
                n95 = Equal?(x=w222, y=w220) -> (x = y?=w219:bool)
              }
              n96 = Or Array Elements(Boolean array=w199) -> (logical OR=w195:bool)
              n97 = case shown="False" w195 {
                tunnel: w194 -> [w203 w211]
                tunnel: w193 -> [w202 w210]
                tunnel: w192 -> [w201 w209]
                tunnel: [w200 w208] -> w191
                frame True {
                  n98 = in-place {
                    in-place-border: w202 -> [w206]
                    in-place-border: w201 -> [w205]
                    n99 = in-place-cluster #3(w203) -> ("Timing 0"=w207:dbl[])
                    n100 = Build Array (concatenate)(w207, w206, w205) -> (w204:dbl[])
                    n101 = in-place-cluster #3("Timing 0"=w204) -> (w200:cluster{"Timing 0":dbl[]})
                  }
                }
                frame False {
                  n102 = in-place {
                    in-place-border: w210 -> [w215]
                    in-place-border: w209 -> [w214]
                    n103 = in-place-cluster #4(w211) -> ("Timing 0"=w217:dbl[])
                    n104 = Add(x=w215, y=w214) -> (x+y=w213:dbl)
                    n105 = Build Array (concatenate)(w217, 0.0 ("element"), w213) -> (w216:dbl[])
                    n106 = in-place-cluster #4("Timing 0"=w216) -> (w208:cluster{"Timing 0":dbl[]})
                  }
                }
              }
            }
          }
          frame "Linear in Y" {
            n107 = for {
              tunnel: w227 -> [w231] mode=indexing
              tunnel: w226 -> [w233]
              tunnel: w225 -> [w230]
              tunnel: w224 -> [w229]
              tunnel: [w228] -> w223 mode=indexing
              i -> [w234]
              # "Check if the current channel is one of the list"
              n108 = for {
                tunnel: w233 -> [w258]
                tunnel: w234 -> [w257]
                tunnel: [w256] -> w236 mode=indexing
                tunnel: string[] ["LD pump", "LD repump", "pulse Y"] -> [w255] mode=indexing
                n109 = Look In Map(map=w258, key=w255) -> (value=w259:i32)  [unwired: 1 in, 1 out]
                n110 = Equal?(x=w259, y=w257) -> (x = y?=w256:bool)
              }
              n111 = Or Array Elements(Boolean array=w236) -> (logical OR=w232:bool)
              n112 = case shown="True" w232 {
                tunnel: w231 -> [w240 w248]
                tunnel: w230 -> [w239 w247]
                tunnel: w229 -> [w238 w246]
                tunnel: [w237 w245] -> w228
                frame True {
                  n113 = in-place {
                    in-place-border: w239 -> [w243]
                    in-place-border: w238 -> [w242]
                    n114 = in-place-cluster #5(w240) -> ("Timing 0"=w244:dbl[])
                    n115 = Build Array (concatenate)(w244, w243, w242) -> (w241:dbl[])
                    n116 = in-place-cluster #5("Timing 0"=w241) -> (w237:cluster{"Timing 0":dbl[]})
                  }
                }
                frame False {
                  n117 = in-place {
                    in-place-border: w247 -> [w252]
                    in-place-border: w246 -> [w251]
                    n118 = in-place-cluster #6(w248) -> ("Timing 0"=w254:dbl[])
                    n119 = Add(x=w252, y=w251) -> (x+y=w250:dbl)
                    n120 = Build Array (concatenate)(w254, 0.0 ("element"), w250) -> (w253:dbl[])
                    n121 = in-place-cluster #6("Timing 0"=w253) -> (w245:cluster{"Timing 0":dbl[]})
                  }
                }
              }
            }
          }
          frame "Linear in Z" {
            n122 = for {
              tunnel: w264 -> [w268] mode=indexing
              tunnel: w263 -> [w270]
              tunnel: w262 -> [w267]
              tunnel: w261 -> [w266]
              tunnel: [w265] -> w260 mode=indexing
              i -> [w271]
              # "Check if the current channel is one of the list"
              n123 = for {
                tunnel: w270 -> [w295]
                tunnel: w271 -> [w294]
                tunnel: [w293] -> w273 mode=indexing
                tunnel: string[] ["LD pump", "LD repump", "pulse Z"] -> [w292] mode=indexing
                n124 = Look In Map(map=w295, key=w292) -> (value=w296:i32)  [unwired: 1 in, 1 out]
                n125 = Equal?(x=w296, y=w294) -> (x = y?=w293:bool)
              }
              n126 = Or Array Elements(Boolean array=w273) -> (logical OR=w269:bool)
              n127 = case shown="True" w269 {
                tunnel: w268 -> [w277 w285]
                tunnel: w267 -> [w276 w284]
                tunnel: w266 -> [w275 w283]
                tunnel: [w274 w282] -> w265
                frame True {
                  n128 = in-place {
                    in-place-border: w276 -> [w280]
                    in-place-border: w275 -> [w279]
                    n129 = in-place-cluster #7(w277) -> ("Timing 0"=w281:dbl[])
                    n130 = Build Array (concatenate)(w281, w280, w279) -> (w278:dbl[])
                    n131 = in-place-cluster #7("Timing 0"=w278) -> (w274:cluster{"Timing 0":dbl[]})
                  }
                }
                frame False {
                  n132 = in-place {
                    in-place-border: w284 -> [w289]
                    in-place-border: w283 -> [w288]
                    n133 = in-place-cluster #8(w285) -> ("Timing 0"=w291:dbl[])
                    n134 = Add(x=w289, y=w288) -> (x+y=w287:dbl)
                    n135 = Build Array (concatenate)(w291, 0.0 ("element"), w287) -> (w290:dbl[])
                    n136 = in-place-cluster #8("Timing 0"=w290) -> (w282:cluster{"Timing 0":dbl[]})
                  }
                }
              }
            }
          }
        }
      }
      event "Run single FID", "Run single FID 2": Mouse Down {
        w319 = "\\temp_multi_FID\\" ("string")
        n137 = event-data() -> ()  [unwired: 1 in, 8 out]
        n138 = local read "Resource Address"() -> (w332:T3)
        n139 = local read "Config folder"() -> (w316:string)
        n140 = local read "Multi-FID"() -> (w317:bool)
        n141 = flat-sequence {
          tunnel: w326 -> [w484]
          tunnel: [w483] -> w325
          frame #0 {
            n142 = Wait (ms)(milliseconds to wait=u32 150) -> ()  [unwired: 1 out]
          }
          frame #1 {
            n143 = invoke on="Run single FID" class="Bool (strict)" method="Reinit To Default"(error in=w484) -> (error out=w483:errorcluster)  [unwired: 2 in, 2 out]
            n144 = local write "Tab Control"(T8."Run single FID" ("Tab Control")) -> ()
          }
        }
        n145 = Concatenate Strings("Config_files\\" ("string"), w316, w319) -> (w320:string)
        n146 = case shown="True" w317 {
          tunnel: w320 -> [_ w337]
          tunnel: [w333 w336] -> w322
          tunnel: w316 -> [_ _]
          frame False {
            n147 = Concatenate Strings("\\pulse_sequence_DAQ.ini" ("string")) -> (w334:string)
            n148 = Build Array(w334) -> (w333:string[])
          }
          frame True {
            n149 = call <vilib>:"Application Directory.vi"() -> ("Application Directory"=w338:path)
            n150 = Build Path(base path=w338, name or relative path=w337) -> (appended path=w339:path)
            n151 = List Folder(path=w339) -> (filenames=w336:string[])  [unwired: 3 in, 3 out]
          }
        }
        n152 = Concatenate Strings(w316, w319) -> (w318:string)
        n153 = Concatenate Strings(w316, "\\Zurich_params.ini" ("string")) -> (w328:string)
        n154 = Concatenate Strings(w316, "\\Keithley_params.ini" ("string")) -> (w329:string)
        n155 = for {
          tunnel: w332 -> [w401]
          tunnel: w329 -> [w397]
          tunnel: w328 -> [w396]
          shift-right: [w359] -> w323
          shift-left: w325 -> [w389]
          tunnel: w322 -> [w344] mode=indexing
          tunnel: w318 -> [w342]
          tunnel: w317 -> [w341]
          tunnel: w316 -> [w340]
          w363 = T13 {"R"=[], "Theta"=[], "X"=[], "Y"=[], "AuxIn0"=[], "AuxIn1"=[], "Frequency"=[], "DIO"=[], "Time"=[]} ("ZI Data")
          w386 = u16 58000 ("Fixed Number Of Points")
          n156 = property on="Rotation signal" class="XYGraph (strict)"("Visible"=TRUE) -> (error out=w355:errorcluster)  [unwired: 2 in, 1 out]
          n157 = property on="Rotation signal 3" class="XYGraph (strict)"("Visible"=FALSE) -> (error out=w356:errorcluster)  [unwired: 2 in, 1 out]
          n158 = invoke on="A" class="DigNum (strict)" method="Reinit To Default"() -> (error out=w351:errorcluster)  [unwired: 3 in, 2 out]
          n159 = invoke on="B" class="DigNum (strict)" method="Reinit To Default"() -> (error out=w350:errorcluster)  [unwired: 3 in, 2 out]
          n160 = invoke on="C" class="DigNum (strict)" method="Reinit To Default"() -> (error out=w349:errorcluster)  [unwired: 3 in, 2 out]
          n161 = invoke on="g1" class="DigNum (strict)" method="Reinit To Default"() -> (error out=w348:errorcluster)  [unwired: 3 in, 2 out]
          n162 = invoke on="g2" class="DigNum (strict)" method="Reinit To Default"() -> (error out=w352:errorcluster)  [unwired: 3 in, 2 out]
          n163 = invoke on="w" class="DigNum (strict)" method="Reinit To Default"() -> (error out=w353:errorcluster)  [unwired: 3 in, 2 out]
          n164 = invoke on="q" class="DigNum (strict)" method="Reinit To Default"() -> (error out=w354:errorcluster)  [unwired: 3 in, 2 out]
          n165 = case shown="False" w341 {
            tunnel: w344 -> [w404 w407]
            tunnel: [w402 w406] -> w343
            tunnel: w342 -> [_ w405]
            tunnel: w340 -> [w403 _]
            frame False {
              n166 = Concatenate Strings(w403, w404) -> (w402:string)
            }
            frame True {
              n167 = Concatenate Strings(w405, w407) -> (w406:string)
            }
          }
          n168 = Bundle By Name(cluster=T7 {"ZI config file (.ini)"="Config_Ver_2\\Zurich_params.ini", "Keithley config file (.ini)"="Config_Ver_2\\Keithley_params.ini", "DAQ config file (.ini)"="Config_Ver_2\\pulse_sequence_DAQ.ini"} ("Config files paths"), "ZI config file (.ini)"=w396, "Keithley config file (.ini)"=w397, "DAQ config file (.ini)"=w343) -> (w393:T7)
          n169 = Build Array(w363, w363) -> (w362:T13[])
          n170 = call "Initialize_Devices_Main_v2.vi"("error in"=w389, "Resource Address"=w401) -> ("error out"=w399:errorcluster, "Resources"=w400:T14)  [unwired: 8 in]
          n171 = Merge Errors(w351, w350, w349, w348, w352, w353, w354, w355, w356) -> (w345:errorcluster)
          n172 = Obtain Queue(name (unnamed)="Data Queue", element data type=w362, error in (no error)=w389) -> (queue out=w388:refnum<queue>, error out=w365:errorcluster)  [unwired: 2 in, 1 out]
          n173 = call "Configurate_All_Main_v2.vi"("Resources in"=w400, "Config files paths"=w393, "error in"=w399) -> ("Resources out"=w395:T14, "error out"=w394:errorcluster)  [unwired: 6 in, 5 out]
          n174 = for {
            N: "Number of repetition" -> [w460]
            tunnel: w393 -> [w465]
            shift-right: [w464] -> w392
            shift-left: w395 -> [w467]
            shift-right: [w452] -> w391
            shift-left: w394 -> [w466]
            tunnel: w388 -> [w455]
            i -> [w461]
            n175 = Divide(x=w461, y=w460) -> (x/y=w458:dbl)
            n176 = call "Single_Measurement_Main_v2.vi"("Config files paths"=w465, "error in"=w466, "Resources in"=w467) -> ("error out"=w462:errorcluster, "Resources out"=w463:T14)  [unwired: 6 in, 1 out]
            n177 = Multiply(x=w458, y=100.0) -> (x*y=→"Progress":dbl)
            n178 = call "Poll_Data_Main_v2.vi"("error in"=w462, "Resources in"=w463) -> ("error out"=w453:errorcluster, "ZI Data 3"=w454:T13, "ZI Data 0"=w451:T13, "Resources out"=w464:T14)  [unwired: 6 in]
            n179 = Build Array(w451, w454) -> (w456:T13[])
            n180 = Enqueue Element(queue=w455, element=w456, error in (no error)=w453) -> (error out=w452:errorcluster)  [unwired: 1 in, 2 out]
          }
          n181 = Initialize Array(0.0 ("element"), w386) -> (w384:dbl[])
          n182 = Merge Errors(w365, w345) -> (w364:errorcluster)
          n183 = for {
            N: "Number of repetition" -> [_]
            tunnel: w388 -> [w444]
            shift-right: [w441] -> w361
            shift-left: w364 -> [w446]
            tunnel: [w444] -> w387
            shift-right: [w434] -> w369
            shift-left: w384 -> [w437]
            tunnel: w386 -> [w440]
            shift-right: [w435] -> w370
            shift-left: w384 -> [w436]
            tunnel: [w423] -> w383
            tunnel: ["Signal in X or Y (?)"] -> w382
            n184 = Dequeue Element(queue=w444, timeout in ms (-1)=10000, error in (no error)=w446) -> (element=w445:T13[], error out=w442:errorcluster)  [unwired: 2 out]
            n185 = Index Array(array=w445) -> (element #1=w425:T13, element #2=w443:T13)  [unwired: 2 in]
            n186 = call "Clear_Data_Main_v2.vi"("ZI Data 0"=w425, "ZI Data 3"=w443, "Time Of Collected Data (ms)"=500.0, 3:"Fixed Number Of Points"=w440, "error in"=w442, 10:"Fixed Number Of Points"=TRUE ("Fixed Number Of Points"), "Check Phase Mismatch"=FALSE) -> ("Cutted Data 0"=w439:T17, "Cutted Data 3"=w438:T17, "error out"=w441:errorcluster)  [unwired: 7 in, 3 out]
            n187 = call "Prepare_plots_SubVI_v1.vi"("Signal in X or Y (?)"="Signal in X or Y (?)", "Y rot avg in"=w436, "X rot avg in"=w437, "Cutted Data 3"=w438, "Cutted Data 0"=w439) -> ("Y rot avg out"=w435:dbl[], "X rot avg out"=w434:dbl[], "Monitor"=→"Intensity signal":cluster{"Time":dbl[], dbl[]}, "RF out"=→"Differential signal":cluster{"Time":dbl[], "Y":dbl[]}[], "Rotation spectrum"=→"Rotation spectrum":waveform(dbl)[], "Rotation"=w430:cluster{"Time":dbl[], dbl[]}[], "Polarimeter"=→"Polarimeter":dbl)
            n188 = Index Array(array=w430) -> (element #1=w429:cluster{"Time":dbl[], dbl[]}, element #2=w428:cluster{"Time":dbl[], dbl[]})  [unwired: 2 in]
            n189 = Select(t=w429, s="Signal in X or Y (?)", f=w428) -> (s? t:f=w423:cluster{"Time":dbl[], dbl[]})
            "Rotation signal" <- w423
          }
          n190 = call "Close_Devices_Main_v2.vi"("error in"=w391, "Resources"=w392) -> ("error out"=w371:errorcluster)  [unwired: 9 in]
          n191 = flat-sequence {
            tunnel: w371 -> [_]
            frame #0 {
              n192 = local write "Progress"(100.0 ("Progress")) -> ()
            }
          }
          n193 = Merge Errors(w371, w361) -> (w360:errorcluster)
          n194 = Divide(x=w369, y="Number of repetition") -> (x/y=w367:dbl[])
          n195 = Divide(x=w370, y="Number of repetition") -> (x/y=w368:dbl[])
          n196 = Unbundle By Name(w383) -> ("Time"=w374:dbl[])
          n197 = Release Queue(queue=w387, error in (no error)=w360) -> (error out=w359:errorcluster)  [unwired: 1 in, 2 out]
          n198 = Build Array(w367, w368) -> (w375:dbl[][])
          n199 = Bundle("Time"=w374, w367) -> (w380:cluster{"Time":dbl[], dbl[]})  [unwired: 1 in]
          n200 = Bundle("Time"=w374, w368) -> (w381:cluster{"Time":dbl[], dbl[]})  [unwired: 1 in]
          n201 = Index Array(array=w374, index #1=1 ("index"), index #2=0 ("index")) -> (element #1=w378:dbl, element #2=w379:dbl)
          n202 = Select(t=w380, s=w382, f=w381) -> (s? t:f=w357:cluster{"Time":dbl[], dbl[]})
          n203 = Subtract(x=w378, y=w379) -> (x-y=w373:dbl)
          n204 = local write "Rotation signal"(w357) -> ()
          n205 = local read "save"() -> (w358:bool)
          n206 = for {
            tunnel: w375 -> [w422] mode=indexing
            tunnel: [w420] -> w372 mode=indexing
            tunnel: w373 -> [w417]
            n207 = call <vilib>:"Auto Power Spectrum.vi"("dt"=w417, "Signal (V)"=w422) -> ("df"=w421:dbl, "Power Spectrum (V^2 rms)"=w419:dbl[])
            n208 = Square Root(x=w419) -> (sqrt(x)=w418:dbl[])
            n209 = Bundle By Name("Y"=w418, "dt"=w421) -> (w420:waveform(dbl))  [unwired: 1 in]
          }
          n210 = case shown="True" w358 {
            tunnel: w357 -> [_ w416]
            frame False {
            }
            frame True {
              n211 = Unbundle(w416) -> ("Time"=w415:dbl[], w414:dbl[])
              n212 = Build Array(w415, w414) -> (w413:dbl[][])
              n213 = call <vilib>:"Create File with Incrementing Suffix.vi"("format string (\" (%d)\")"=" %d" ("format string (\" (%d)\")"), "file path"=path "C:/Users/Daniel/Desktop/tests/test.dat") -> ("actual path"=w410:path)  [unwired: 7 in, 2 out]
              n214 = Transpose 2D Array(2D array=w413) -> (transposed array=w412:dbl[][])
              n215 = call-poly <vilib>:"Write Delimited Spreadsheet.vi"("file path (dialog if empty)"=w410, "format (%.3f)"="%.6f", "2D data"=w412) -> ()  [unwired: 11 in, 2 out]
            }
          }
          n216 = local write "Rotation spectrum"(w372) -> ()
        }
        n217 = case shown="Error .." w323 {
          selector: w323 -> [w468 w469]
          tunnel: [w468 w472] -> w324
          frame No Error {
          }
          frame Error {
            w477 = "\r\n"
            n218 = Unbundle By Name(w469) -> ("code"=w480:i32, "source"=w478:string)
            n219 = Number To Decimal String(number=w480) -> (decimal integer string=w479:string)  [unwired: 1 in]
            n220 = Concatenate Strings("There is an error:" ("string"), w477, w479, w477, w478, w477, "Do you want to clear it?" ("string")) -> (w473:string)
            n221 = Two Button Dialog(message=w473, 1:"No" ("F button name (\"Cancel\")"), 2:"Yes" ("T button name (\"OK\")")) -> (T button?=w471:bool)
            n222 = call <vilib>:"Clear Errors.vi"("error in (no error)"=w469) -> ("error out"=w470:errorcluster)  [unwired: 5 in, 1 out]
            n223 = Select(t=w470, s=w471, f=w469) -> (s? t:f=w472:errorcluster)
          }
        }
      }
      event "Run tomography", "Run tomography 2": Mouse Down {
        w494 = T13 {"R"=[], "Theta"=[], "X"=[], "Y"=[], "AuxIn0"=[], "AuxIn1"=[], "Frequency"=[], "DIO"=[], "Time"=[]} ("ZI Data")
        w489 = "\\tomography" ("string")
        n224 = event-data() -> ()  [unwired: 1 in, 8 out]
        n225 = local read "Config folder"() -> (w490:string)
        n226 = local read "Resource Address"() -> (w519:T3)
        n227 = Build Array(w494, w494) -> (w493:T13[])
        n228 = flat-sequence {
          frame #0 {
            n229 = Wait (ms)(milliseconds to wait=u32 150) -> ()  [unwired: 1 out]
          }
          frame #1 {
            n230 = invoke on="Run tomography" class="Bool (strict)" method="Reinit To Default"() -> ()  [unwired: 3 in, 3 out]
            n231 = local write "Tab Control"(T10."Run tomography" ("Tab Control")) -> ()
          }
        }
        n232 = Concatenate Strings("Config_files\\" ("string"), w490, w489) -> (w492:string)
        n233 = Concatenate Strings(w490, w489, "\\" ("string")) -> (w488:string)
        n234 = call <vilib>:"Application Directory.vi"() -> ("Application Directory"=w522:path)
        n235 = Obtain Queue(name (unnamed)="Data Queue 2", element data type=w493, error in (no error)=w514) -> (queue out=w516:refnum<queue>, error out=w513:errorcluster)  [unwired: 2 in, 1 out]
        n236 = property on="Plot type" class="Ring (strict)"("DisabledEnum"=T9."Disabled and Grayed Out" ("Disabled")) -> (error out=w500:errorcluster)  [unwired: 2 in, 1 out]
        n237 = Concatenate Strings(w490, "\\Zurich_params.ini" ("string")) -> (w525:string)
        n238 = Concatenate Strings(w490, "\\Keithley_params.ini" ("string")) -> (w526:string)
        n239 = Build Path(base path=w522, name or relative path=w492) -> (appended path=w523:path)
        n240 = List Folder(path=w523) -> (filenames=w521:string[])  [unwired: 3 in, 3 out]
        n241 = call "Initialize_Devices_Main_v2.vi"("error in"=w513, "Resource Address"=w519) -> ("error out"=w517:errorcluster, "Resources"=w518:T14)  [unwired: 8 in]
        n242 = for {
          tunnel: "pulses type (priv)" -> [w532] mode=indexing
          tunnel: [w530] -> w503 mode=concatenating
          n243 = for {
            tunnel: " + " ("string") -> [w537]
            tunnel: w532 -> [w536]
            tunnel: string[] ["[ None ]", "[ Y pi ]", "[ Z(pi/2)+Y(pi) ]"] -> [w535] mode=indexing
            tunnel: [w534] -> w530 mode=indexing
            n244 = Concatenate Strings(w536, w537, w535) -> (w534:string)
          }
        }
        n245 = for {
          N -> [w566]
          tunnel: w526 -> [w574]
          tunnel: w525 -> [w573]
          tunnel: w521 -> [w538] mode=indexing
          shift-right: [w569] -> w486
          shift-left: w517 -> [w544]
          tunnel: w516 -> [w570]
          shift-right: [w571] -> w512
          shift-left: w518 -> [w543]
          tunnel: u16 58000 ("Fixed Number Of Points") -> [w567]
          tunnel: [w568] -> w510
          shift-right: [w562] -> w507
          shift-left: dbl[][] [] -> [w563]
          tunnel: w503 -> [_]
          tunnel: [w559] -> w502 mode=indexing
          tunnel: w500 -> [_]
          tunnel: w488 -> [w540]
          i -> [w560]
          n246 = Concatenate Strings(w540, w538) -> (w539:string)
          n247 = Multiply(x="Averaging", y=w560) -> (x*y=w565:i32)
          n248 = Bundle By Name(cluster=T7 {"ZI config file (.ini)"="Config_Ver_2\\Zurich_params.ini", "Keithley config file (.ini)"="Config_Ver_2\\Keithley_params.ini", "DAQ config file (.ini)"="Config_Ver_2\\pulse_sequence_DAQ.ini"} ("Config files paths"), "ZI config file (.ini)"=w573, "Keithley config file (.ini)"=w574, "DAQ config file (.ini)"=w539) -> (w541:T7)
          n249 = call "Configurate_All_Main_v2.vi"("Resources in"=w543, "Config files paths"=w541, "error in"=w544) -> ("Resources out"=w542:T14, "error out"=w545:errorcluster)  [unwired: 6 in, 5 out]
          n250 = for {
            N: "Averaging" -> [w623]
            shift-right: [w635] -> w571
            shift-left: w542 -> [w637]
            shift-right: [w626] -> w557
            shift-left: w545 -> [w636]
            tunnel: w570 -> [w628]
            tunnel: w541 -> [w625]
            tunnel: w566 -> [w624]
            tunnel: w565 -> [w620]
            i -> [w621]
            n251 = Add(x=w621, y=w620) -> (x+y=w619:i32)
            n252 = Multiply(x=w623, y=w624) -> (x*y=w622:i32)
            n253 = call "Single_Measurement_Main_v2.vi"("Config files paths"=w625, "error in"=w636, "Resources in"=w637) -> ("error out"=w633:errorcluster, "Resources out"=w634:T14)  [unwired: 6 in, 1 out]
            n254 = call "Poll_Data_Main_v2.vi"("error in"=w633, "Resources in"=w634) -> ("error out"=w627:errorcluster, "ZI Data 3"=w630:T13, "ZI Data 0"=w617:T13, "Resources out"=w635:T14)  [unwired: 6 in]
            n255 = Divide(x=w619, y=w622) -> (x/y=w631:dbl)
            n256 = Build Array(w617, w630) -> (w629:T13[])
            n257 = Multiply(x=w631, y=100.0) -> (x*y=→"Progress":dbl)
            n258 = Enqueue Element(queue=w628, element=w629, error in (no error)=w627) -> (error out=w626:errorcluster)  [unwired: 1 in, 2 out]
          }
          n259 = Initialize Array(0.0 ("element"), w567) -> (w554:dbl[])
          n260 = for {
            N: "Averaging" -> [_]
            shift-right: [w608] -> w558
            shift-left: w544 -> [w613]
            shift-right: [w602] -> w552
            shift-left: w554 -> [w605]
            shift-right: [w603] -> w553
            shift-left: w554 -> [w604]
            tunnel: [w595] -> w548
            tunnel: w570 -> [w594]
            tunnel: w567 -> [w593]
            tunnel: [w592] -> w550
            n261 = local read "Signal in X or Y (?)"() -> (w595:bool)
            n262 = Dequeue Element(queue=w594, timeout in ms (-1)=10000, error in (no error)=w613) -> (element=w612:T13[], error out=w609:errorcluster)  [unwired: 2 out]
            n263 = Index Array(array=w612) -> (element #1=w610:T13, element #2=w611:T13)  [unwired: 2 in]
            n264 = call "Clear_Data_Main_v2.vi"("ZI Data 0"=w610, "ZI Data 3"=w611, "Time Of Collected Data (ms)"=500.0, 3:"Fixed Number Of Points"=w593, "error in"=w609, 10:"Fixed Number Of Points"=TRUE ("Fixed Number Of Points"), "Check Phase Mismatch"=FALSE) -> ("Cutted Data 0"=w607:T17, "Cutted Data 3"=w606:T17, "error out"=w608:errorcluster)  [unwired: 7 in, 3 out]
            n265 = call "Prepare_plots_SubVI_v1.vi"("Signal in X or Y (?)"=w595, "Y rot avg in"=w604, "X rot avg in"=w605, "Cutted Data 3"=w606, "Cutted Data 0"=w607) -> ("Y rot avg out"=w603:dbl[], "X rot avg out"=w602:dbl[], "Monitor"=→"Intensity signal":cluster{"Time":dbl[], dbl[]}, "RF out"=→"Differential signal":cluster{"Time":dbl[], "Y":dbl[]}[], "Rotation spectrum"=→"Rotation spectrum":waveform(dbl)[], "Rotation"=w599:cluster{"Time":dbl[], dbl[]}[])  [unwired: 1 out]
            n266 = Index Array(array=w599) -> (element #1=w598:cluster{"Time":dbl[], dbl[]}, element #2=w597:cluster{"Time":dbl[], dbl[]})  [unwired: 2 in]
            n267 = Select(t=w598, s=w595, f=w597) -> (s? t:f=w592:cluster{"Time":dbl[], dbl[]})
            "Rotation signal" <- w592
          }
          n268 = Divide(x=w552, y="Averaging") -> (x/y=w546:dbl[])
          n269 = Divide(x=w553, y="Averaging") -> (x/y=w547:dbl[])
          n270 = Empty Array?(array=w563) -> (empty?=w551:bool)
          n271 = Unbundle By Name(w550) -> ("Time"=w549:dbl[])
          n272 = Merge Errors(w557, w558) -> (w556:errorcluster)
          n273 = case shown="True" w551 {
            tunnel: w549 -> [w576 w583]
            tunnel: w563 -> [w582 w590]
            tunnel: [w581 w589] -> w562
            tunnel: w548 -> [w580 w588]
            tunnel: w547 -> [w579 w587]
            tunnel: w546 -> [w578 w586]
            tunnel: [w575 w585] -> w561
            frame True {
              n274 = Select(t=w578, s=w580, f=w579) -> (s? t:f=w577:dbl[])
              n275 = Bundle("Time"=w576, w577) -> (w575:cluster{"Time":dbl[], dbl[]})  [unwired: 1 in]
              n276 = Build Array (concatenate)(w582, w576, w577) -> (w581:dbl[][])
            }
            frame False {
              n277 = Select(t=w586, s=w588, f=w587) -> (s? t:f=w584:dbl[])
              n278 = Bundle("Time"=w583, w584) -> (w585:cluster{"Time":dbl[], dbl[]})  [unwired: 1 in]
              n279 = Build Array (concatenate)(w590, w584) -> (w589:dbl[][])
            }
          }
          n280 = Flush Queue(queue=w570, error in (no error)=w556) -> (queue out=w568:refnum<queue>, error out=w569:errorcluster)  [unwired: 1 out]
          n281 = flat-sequence {
            tunnel: w561 -> [w638]
            tunnel: w560 -> [w639]
            tunnel: [w638] -> w559
            frame #0 {
              n282 = local write "Plot type"(w639) -> ()
              "Rotation" <- w638
            }
          }
        }
        "tomography rotation memory (priv)" <- w502
        n283 = property on="Plot type" class="Ring (strict)"("Strings []"=w503) -> ()  [unwired: 2 in, 2 out]
        n284 = Release Queue(queue=w510, error in (no error)=w486) -> (error out=w509:errorcluster)  [unwired: 1 in, 2 out]
        n285 = flat-sequence {
          tunnel: w486 -> [_]
          frame #0 {
            n286 = local write "Progress"(100.0 ("Progress")) -> ()
          }
        }
        n287 = call "Close_Devices_Main_v2.vi"("error in"=w509, "Resources"=w512) -> ("error out"=w498:errorcluster)  [unwired: 9 in]
        n288 = property on="Plot type" class="Ring (strict)"(error in=w486, "DisabledEnum"=T9."Enabled" ("Disabled")) -> (error out=w497:errorcluster)  [unwired: 1 in, 1 out]
        n289 = call "Save_Tomography_Data_Main_v2.vi"("error in"=w486, "Save CYCLOPS data (?)"="Save CYCLOPS data (?)", "Save raw data (?)"="Save raw data (?)", "Data Raw"=w507) -> ("error out"=w496:errorcluster)  [unwired: 6 in, 1 out]
        n290 = Merge Errors(w498, w497, w496) -> (w495:errorcluster)
        n291 = case shown="Error .." w495 {
          selector: w495 -> [w640 w641]
          tunnel: [w640 w644] -> w524
          frame No Error {
          }
          frame Error {
            w649 = "\r\n"
            n292 = Unbundle By Name(w641) -> ("code"=w652:i32, "source"=w650:string)
            n293 = Number To Decimal String(number=w652) -> (decimal integer string=w651:string)  [unwired: 1 in]
            n294 = Concatenate Strings("There is an error:" ("string"), w649, w651, w649, w650, w649, "Do you want to clear it?" ("string")) -> (w645:string)
            n295 = Two Button Dialog(message=w645, 1:"No" ("F button name (\"Cancel\")"), 2:"Yes" ("T button name (\"OK\")")) -> (T button?=w643:bool)
            n296 = call <vilib>:"Clear Errors.vi"("error in (no error)"=w641) -> ("error out"=w642:errorcluster)  [unwired: 5 in, 1 out]
            n297 = Select(t=w642, s=w643, f=w641) -> (s? t:f=w644:errorcluster)
          }
        }
      }
      event "Run QPT", "Run QPT 2": Mouse Down {
        w665 = "\\process\\temp_states" ("string")
        # "9 FIDs compose 1 Tomography"
        n298 = event-data() -> ()  [unwired: 1 in, 8 out]
        n299 = local read "Config folder"() -> (w666:string)
        n300 = local read "Resource Address"() -> (w658:T3)
        n301 = flat-sequence {
          frame #0 {
            n302 = Wait (ms)(milliseconds to wait=u32 150) -> ()  [unwired: 1 out]
          }
          frame #1 {
            n303 = invoke on="Run tomography" class="Bool (strict)" method="Reinit To Default"() -> ()  [unwired: 3 in, 3 out]
            n304 = local write "Tab Control"(T1."Run QPT" ("Tab Control")) -> ()
          }
        }
        n305 = Concatenate Strings("Config_files\\" ("string"), w666, w665) -> (w668:string)
        n306 = Concatenate Strings(w666, w665, "\\" ("string")) -> (w664:string)
        n307 = call <vilib>:"Application Directory.vi"() -> ("Application Directory"=w676:path)
        n308 = property on="Plot type" class="Ring (strict)"("DisabledEnum"=T9."Disabled and Grayed Out" ("Disabled")) -> (error out=w662:errorcluster)  [unwired: 2 in, 1 out]
        n309 = Concatenate Strings(w666, "\\Zurich_params.ini" ("string")) -> (w679:string)
        n310 = Concatenate Strings(w666, "\\Keithley_params.ini" ("string")) -> (w680:string)
        n311 = Build Path(base path=w676, name or relative path=w668) -> (appended path=w677:path)
        n312 = List Folder(path=w677) -> (filenames=w661:string[])  [unwired: 3 in, 3 out]
        n313 = call "Splitting_filename.vi"("Splitting number"=u32 9, "Total filenames"=w661) -> ("Splitted filenames"=w660:string[][])  [unwired: 9 in]
        n314 = for {
          N -> [w707]
          tunnel: w680 -> [w718]
          tunnel: w679 -> [w717]
          tunnel: "Save CYCLOPS data (?) 2" -> [w687]
          tunnel: "Save raw data (?) 2" -> [w688]
          tunnel: w664 -> [w714]
          tunnel: w660 -> [w713] mode=indexing
          shift-right: [w715] -> w671
          shift-left: _ -> [_]
          shift-right: [w685] -> w670
          shift-left: w662 -> [w712]
          tunnel: w658 -> [w703]
          tunnel: w657 -> [w700]
          tunnel: [w692] -> w656
          i -> [w690]
          w697 = T13 {"R"=[], "Theta"=[], "X"=[], "Y"=[], "AuxIn0"=[], "AuxIn1"=[], "Frequency"=[], "DIO"=[], "Time"=[]} ("ZI Data")
          n315 = Increment(x=w690) -> (x+1=→"Current_QPT_order":i32)
          n316 = Build Array(w697, w697) -> (w696:T13[])
          n317 = Divide(x=w690, y=w707) -> (x/y=w706:dbl)
          n318 = Multiply(x=100.0, y=w706) -> (x*y=→"QPT Progress":dbl)
          n319 = Obtain Queue(name (unnamed)="Data Queue 2", element data type=w696, error in (no error)=w700) -> (queue out=w699:refnum<queue>, error out=w698:errorcluster)  [unwired: 2 in, 1 out]
          n320 = call "Initialize_Devices_Main_v2.vi"("error in"=w698, "Resource Address"=w703) -> ("error out"=w702:errorcluster, "Resources"=w701:T14)  [unwired: 8 in]
          n321 = for {
            N -> [w749]
            tunnel: w718 -> [w756]
            tunnel: w717 -> [w755]
            tunnel: w713 -> [w721] mode=indexing
            shift-right: [w752] -> w686
            shift-left: w702 -> [w727]
            shift-right: [w753] -> w693
            shift-left: w701 -> [w726]
            tunnel: u16 58000 ("Fixed Number Of Points") -> [w750]
            tunnel: [w751] -> w711
            shift-right: [w745] -> w689
            shift-left: dbl[][] [] -> [w746]
            tunnel: [w742] -> w708 mode=indexing
            tunnel: w714 -> [w723]
            tunnel: w712 -> [_]
            tunnel: w699 -> [w720]
            i -> [w743]
            n322 = Concatenate Strings(w723, w721) -> (w722:string)
            n323 = Multiply(x="Averaging 2", y=w743) -> (x*y=w748:i32)
            n324 = Bundle By Name(cluster=T7 {"ZI config file (.ini)"="Config_Ver_2\\Zurich_params.ini", "Keithley config file (.ini)"="Config_Ver_2\\Keithley_params.ini", "DAQ config file (.ini)"="Config_Ver_2\\pulse_sequence_DAQ.ini"} ("Config files paths"), "ZI config file (.ini)"=w755, "Keithley config file (.ini)"=w756, "DAQ config file (.ini)"=w722) -> (w724:T7)
            n325 = call "Configurate_All_Main_v2.vi"("Resources in"=w726, "Config files paths"=w724, "error in"=w727) -> ("Resources out"=w725:T14, "error out"=w728:errorcluster)  [unwired: 6 in, 5 out]
            n326 = for {
              N: "Averaging 2" -> [w805]
              shift-right: [w817] -> w753
              shift-left: w725 -> [w819]
              shift-right: [w808] -> w740
              shift-left: w728 -> [w818]
              tunnel: w720 -> [w810]
              tunnel: w724 -> [w807]
              tunnel: w749 -> [w806]
              tunnel: w748 -> [w802]
              i -> [w803]
              n327 = Add(x=w803, y=w802) -> (x+y=w801:i32)
              n328 = Multiply(x=w805, y=w806) -> (x*y=w804:i32)
              n329 = call "Single_Measurement_Main_v2.vi"("Config files paths"=w807, "error in"=w818, "Resources in"=w819) -> ("error out"=w815:errorcluster, "Resources out"=w816:T14)  [unwired: 6 in, 1 out]
              n330 = call "Poll_Data_Main_v2.vi"("error in"=w815, "Resources in"=w816) -> ("error out"=w809:errorcluster, "ZI Data 3"=w812:T13, "ZI Data 0"=w799:T13, "Resources out"=w817:T14)  [unwired: 6 in]
              n331 = Divide(x=w801, y=w804) -> (x/y=w813:dbl)
              n332 = Build Array(w799, w812) -> (w811:T13[])
              n333 = Multiply(x=w813, y=100.0) -> (x*y=→"Single Tomography Progress":dbl)
              n334 = Enqueue Element(queue=w810, element=w811, error in (no error)=w809) -> (error out=w808:errorcluster)  [unwired: 1 in, 2 out]
            }
            n335 = Initialize Array(0.0 ("element"), w750) -> (w737:dbl[])
            n336 = for {
              N: "Averaging 2" -> [_]
              shift-right: [w790] -> w741
              shift-left: w727 -> [w795]
              shift-right: [w784] -> w735
              shift-left: w737 -> [w787]
              shift-right: [w785] -> w736
              shift-left: w737 -> [w786]
              tunnel: [w777] -> w731
              tunnel: w720 -> [w776]
              tunnel: w750 -> [w775]
              tunnel: [w774] -> w733
              n337 = local read "Signal in X or Y (?)"() -> (w777:bool)
              n338 = Dequeue Element(queue=w776, timeout in ms (-1)=10000, error in (no error)=w795) -> (element=w794:T13[], error out=w791:errorcluster)  [unwired: 2 out]
              n339 = Index Array(array=w794) -> (element #1=w792:T13, element #2=w793:T13)  [unwired: 2 in]
              n340 = call "Clear_Data_Main_v2.vi"("ZI Data 0"=w792, "ZI Data 3"=w793, "Time Of Collected Data (ms)"=500.0, 3:"Fixed Number Of Points"=w775, "error in"=w791, 10:"Fixed Number Of Points"=TRUE ("Fixed Number Of Points"), "Check Phase Mismatch"=FALSE) -> ("Cutted Data 0"=w789:T17, "Cutted Data 3"=w788:T17, "error out"=w790:errorcluster)  [unwired: 7 in, 3 out]
              n341 = call "Prepare_plots_SubVI_v1.vi"("Signal in X or Y (?)"=w777, "Y rot avg in"=w786, "X rot avg in"=w787, "Cutted Data 3"=w788, "Cutted Data 0"=w789) -> ("Y rot avg out"=w785:dbl[], "X rot avg out"=w784:dbl[], "Monitor"=→"Intensity signal 2":cluster{"Time":dbl[], dbl[]}, "RF out"=→"Differential signal 2":cluster{"Time":dbl[], "Y":dbl[]}[], "Rotation spectrum"=→"Rotation spectrum 2":waveform(dbl)[], "Rotation"=w781:cluster{"Time":dbl[], dbl[]}[])  [unwired: 1 out]
              n342 = Index Array(array=w781) -> (element #1=w780:cluster{"Time":dbl[], dbl[]}, element #2=w779:cluster{"Time":dbl[], dbl[]})  [unwired: 2 in]
              n343 = Select(t=w780, s=w777, f=w779) -> (s? t:f=w774:cluster{"Time":dbl[], dbl[]})
              "Rotation signal 2" <- w774
            }
            n344 = Divide(x=w735, y="Averaging 2") -> (x/y=w729:dbl[])
            n345 = Divide(x=w736, y="Averaging 2") -> (x/y=w730:dbl[])
            n346 = Empty Array?(array=w746) -> (empty?=w734:bool)
            n347 = Unbundle By Name(w733) -> ("Time"=w732:dbl[])
            n348 = Merge Errors(w740, w741) -> (w739:errorcluster)
            n349 = case shown="True" w734 {
              tunnel: w732 -> [w758 w765]
              tunnel: w746 -> [w764 w772]
              tunnel: [w763 w771] -> w745
              tunnel: w731 -> [w762 w770]
              tunnel: w730 -> [w761 w769]
              tunnel: w729 -> [w760 w768]
              tunnel: [w757 w767] -> w744
              frame True {
                n350 = Select(t=w760, s=w762, f=w761) -> (s? t:f=w759:dbl[])
                n351 = Bundle("Time"=w758, w759) -> (w757:cluster{"Time":dbl[], dbl[]})  [unwired: 1 in]
                n352 = Build Array (concatenate)(w764, w758, w759) -> (w763:dbl[][])
              }
              frame False {
                n353 = Select(t=w768, s=w770, f=w769) -> (s? t:f=w766:dbl[])
                n354 = Bundle("Time"=w765, w766) -> (w767:cluster{"Time":dbl[], dbl[]})  [unwired: 1 in]
                n355 = Build Array (concatenate)(w772, w766) -> (w771:dbl[][])
              }
            }
            n356 = Flush Queue(queue=w720, error in (no error)=w739) -> (queue out=w751:refnum<queue>, error out=w752:errorcluster)  [unwired: 1 out]
            n357 = flat-sequence {
              tunnel: w744 -> [w820]
              tunnel: w743 -> [w821]
              tunnel: [w820] -> w742
              frame #0 {
                n358 = local write "Plot type"(w821) -> ()
                "Rotation 2" <- w820
              }
            }
          }
          "tomography rotation memory (priv) 2" <- w708
          n359 = local read "Current_QPT_order"() -> (w684:i32)
          n360 = Release Queue(queue=w711, error in (no error)=w686) -> (error out=w694:errorcluster)  [unwired: 1 in, 2 out]
          n361 = flat-sequence {
            tunnel: w686 -> [_]
            frame #0 {
              n362 = local write "Single Tomography Progress"(100.0 ("Progress")) -> ()
            }
          }
          n363 = property on="Plot type" class="Ring (strict)"(error in=w686, "DisabledEnum"=T9."Enabled" ("Disabled")) -> (error out=w715:errorcluster)  [unwired: 1 in, 1 out]
          n364 = call "Save_QPT_Data_Main_v2.vi"("Numeric"=w684, "error in"=w686, "Save CYCLOPS data (?)"=w687, "Save raw data (?)"=w688, "Data Raw"=w689) -> ("error out"=w685:errorcluster)  [unwired: 5 in, 1 out]
          n365 = call "Close_Devices_Main_v2.vi"("error in"=w694, "Resources"=w693) -> ("error out"=w692:errorcluster)  [unwired: 9 in]
        }
        n366 = flat-sequence {
          tunnel: w656 -> [_]
          frame #0 {
            n367 = local write "QPT Progress"(100.0 ("x")) -> ()
          }
        }
        n368 = Merge Errors(w656, w671, w670) -> (w669:errorcluster)
        n369 = case shown="Error .." w669 {
          selector: w669 -> [w822 w823]
          tunnel: [w822 w826] -> w678
          frame No Error {
          }
          frame Error {
            w831 = "\r\n"
            n370 = Unbundle By Name(w823) -> ("code"=w834:i32, "source"=w832:string)
            n371 = Number To Decimal String(number=w834) -> (decimal integer string=w833:string)  [unwired: 1 in]
            n372 = Concatenate Strings("There is an error:" ("string"), w831, w833, w831, w832, w831, "Do you want to clear it?" ("string")) -> (w827:string)
            n373 = Two Button Dialog(message=w827, 1:"No" ("F button name (\"Cancel\")"), 2:"Yes" ("T button name (\"OK\")")) -> (T button?=w825:bool)
            n374 = call <vilib>:"Clear Errors.vi"("error in (no error)"=w823) -> ("error out"=w824:errorcluster)  [unwired: 5 in, 1 out]
            n375 = Select(t=w824, s=w825, f=w823) -> (s? t:f=w826:errorcluster)
          }
        }
      }
      event "Plot type": Value Change {
        n376 = event-data() -> ()  [unwired: 1 in, 6 out]
        n377 = local read "tomography rotation memory (priv)"() -> (w840:cluster{"Time":dbl[], dbl[]}[])
        n378 = local read "Plot type"() -> (w841:u16)
        n379 = Index Array(array=w840, index=w841) -> (element=w842:cluster{"Time":dbl[], dbl[]})
        n380 = local write "Rotation"(w842) -> ()
      }
      event "Fit model": Mouse Down {
        w848 = 2.0 ("x")
        w866 = 5 ("y")
        w873 = 1 ("index")
        # "q"
        # "w"
        # "g"
        # "C"
        # "B"
        # "A"
        # "initial values:"
        n381 = event-data() -> ()  [unwired: 1 in, 8 out]
        n382 = local read "Rotation signal"() -> (w867:cluster{"Time":dbl[], dbl[]})
        n383 = Decrement(x=w873) -> (x-1=w875:i32)
        n384 = Unbundle(w867) -> ("Time"=w874:dbl[], w871:dbl[])
        n385 = property on="Rotation signal" class="XYGraph (strict)"(error in=w881, "Visible"=FALSE) -> (error out=w879:errorcluster)  [unwired: 1 in, 1 out]
        n386 = property on="Rotation signal 3" class="XYGraph (strict)"(error in=w881, "Visible"=TRUE) -> (error out=w880:errorcluster)  [unwired: 1 in, 1 out]
        n387 = local read "Polarimeter"() -> (w856:dbl)
        n388 = Array Size(array=w871) -> (size(s)=w872:i32)
        n389 = Index Array(array=w874, index #1=w873, index #2=w875) -> (element #1=w876:dbl, element #2=w877:dbl)
        n390 = Multiply(x=1100.0, y=6.283185307179586) -> (x*y=w852:dbl)
        n391 = Subtract(x=w876, y=w877) -> (x-y=w865:dbl)
        n392 = Quotient & Remainder(x=w872, y=w866) -> (floor(x/y)=w870:i32)  [unwired: 1 out]
        n393 = Merge Errors(w879, w880) -> (w878:errorcluster)
        n394 = Reshape Array(w871, w870, w866) -> (w869:dbl[][])
        n395 = Multiply(x=w865, y=w866) -> (x*y=w863:dbl)
        n396 = Index Array(array=w869, index (col)=0 ("disabled index (col)")) -> (element=w845:dbl[])  [unwired: 1 in]
        n397 = Array Subset(array=w845, index=0, length=100) -> (w859:dbl[])
        n398 = Array Max & Min(array=w859) -> (max value=w858:dbl, min value=w857:dbl)  [unwired: 2 out]
        n399 = Subtract(x=w858, y=w857) -> (x-y=w849:dbl)
        n400 = Add(x=w858, y=w857) -> (x+y=w850:dbl)
        n401 = Divide(x=w850, y=w848) -> (x/y=w847:dbl)
        n402 = Divide(x=w849, y=w848) -> (x/y=w846:dbl)
        n403 = Array Size(array=w845) -> (size(s)=w864:i32)
        n404 = for {
          N: w864 -> [_]
          tunnel: w863 -> [w889]
          tunnel: [w888] -> w862 mode=indexing
          i -> [w890]
          n405 = Multiply(x=w889, y=w890) -> (x*y=w888:dbl)
        }
        n406 = Multiply(x=w845, y=1000) -> (x*y=w843:dbl[])
        n407 = case shown="\"Full\"" "Enum" {
          tunnel: [w922 w948 w975] -> w884
          tunnel: [w911 w938 w967] -> w882
          tunnel: w878 -> [w911 w938 w967]
          tunnel: w867 -> [w921 w947 w974]
          tunnel: w862 -> [w914 w941 w970]
          tunnel: w847 -> [w920 _ w953]
          tunnel: w856 -> [w919 w946 w952]
          tunnel: 20.0 -> [w918 w945 w951]
          tunnel: w852 -> [_ w932 w950]
          tunnel: 0.0 -> [_ w933 w949]
          tunnel: w846 -> [_ w934 w954]
          tunnel: w843 -> [w915 w942 w971]
          frame "B*Exp(-q2*t)+C" {
            w923 = nan
            n408 = Build Array(w920, w919, w918) -> (w912:dbl[])
            n409 = call-poly <vilib>:"Nonlinear Curve Fit.vi"("Y"=w915, "initial parameters"=w912, "X"=w914, "model description"=T11 {"model"="b*exp(-g2*t)+c", "Parameters"=["b", "c", "g2"], "x"="t"}, "error in (no error)"=w911) -> ("best nonlinear fit"=w913:dbl[], "best fit parameters"=w909:dbl[])  [unwired: 6 in, 3 out]
            n410 = Divide(x=w913, y=1000) -> (x/y=w917:dbl[])
            n411 = Index Array(array=w909) -> (element #1=w908:dbl, element #2=w907:dbl, element #3=w906:dbl)  [unwired: 3 in]
            n412 = Bundle(w914, w917) -> (w905:cluster{dbl[], dbl[]})  [unwired: 1 in]
            n413 = Build Array(w921, w905) -> (w922:cluster{"Time":dbl[], dbl[]}[])
            n414 = local write "A"(w923) -> ()
            n415 = local write "C"(w907) -> ()
            n416 = local write "g2"(w906) -> ()
            n417 = local write "q"(w923) -> ()
            n418 = local write "w"(w923) -> ()
            n419 = local write "g1"(w923) -> ()
            n420 = local write "B"(w908) -> ()
          }
          frame "A*Sin(w*t+q)*Exp(-g1*t)+C" {
            w931 = nan
            n421 = Build Array(w934, w946, w945, w933, w932) -> (w939:dbl[])
            n422 = call-poly <vilib>:"Nonlinear Curve Fit.vi"("Y"=w942, "initial parameters"=w939, "X"=w941, "model description"=T11 {"model"="a*sin(w*t+q)*exp(-g1*t)+c", "Parameters"=["a", "c", "g1", "q", "w"], "x"="t"}, "error in (no error)"=w938) -> ("best nonlinear fit"=w940:dbl[], "best fit parameters"=w936:dbl[])  [unwired: 6 in, 3 out]
            n423 = Divide(x=w940, y=1000) -> (x/y=w944:dbl[])
            n424 = Index Array(array=w936) -> (element #1=w930:dbl, element #2=w929:dbl, element #3=w928:dbl, element #4=w926:dbl, element #5=w927:dbl)  [unwired: 5 in]
            n425 = Bundle(w941, w944) -> (w935:cluster{dbl[], dbl[]})  [unwired: 1 in]
            n426 = Quotient & Remainder(x=w926, y=6.283185307179586) -> (x-y*floor(x/y)=w924:dbl)  [unwired: 1 out]
            n427 = Build Array(w947, w935) -> (w948:cluster{"Time":dbl[], dbl[]}[])
            n428 = local write "g1"(w928) -> ()
            n429 = local write "w"(w927) -> ()
            n430 = local write "A"(w930) -> ()
            n431 = local write "C"(w929) -> ()
            n432 = local write "q"(w924) -> ()
            n433 = local write "B"(w931) -> ()
            n434 = local write "g2"(w931) -> ()
          }
          frame "Full" {
            n435 = Build Array(w954, w953, w952, w951, w951, w950, w949) -> (w968:dbl[])
            n436 = call-poly <vilib>:"Nonlinear Curve Fit.vi"("Y"=w971, "initial parameters"=w968, "X"=w970, "model description"=T11 {"model"="a*sin(w*t+q)*exp(-g1*t)+b*exp(-g2*t)+c", "Parameters"=["a", "b", "c", "g1", "g2", "w", "q"], "x"="t"}, "error in (no error)"=w967) -> ("best nonlinear fit"=w969:dbl[], "best fit parameters"=w958:dbl[])  [unwired: 6 in, 3 out]
            n437 = Divide(x=w969, y=1000) -> (x/y=w973:dbl[])
            n438 = Index Array(array=w958) -> (element #1=w964:dbl, element #2=w960:dbl, element #3=w961:dbl, element #4=w962:dbl, element #5=w963:dbl, element #6=w959:dbl, element #7=w955:dbl)  [unwired: 7 in]
            n439 = Bundle(w970, w973) -> (w965:cluster{dbl[], dbl[]})  [unwired: 1 in]
            n440 = local write "w"(w959) -> ()
            n441 = local write "A"(w964) -> ()
            n442 = local write "B"(w960) -> ()
            n443 = local write "C"(w961) -> ()
            n444 = local write "g1"(w962) -> ()
            n445 = local write "g2"(w963) -> ()
            n446 = Quotient & Remainder(x=w955, y=6.283185307179586) -> (x-y*floor(x/y)=w956:dbl)  [unwired: 1 out]
            n447 = Build Array(w974, w965) -> (w975:cluster{"Time":dbl[], dbl[]}[])
            n448 = local write "q"(w956) -> ()
          }
        }
        n449 = Reverse 1D Array(array=w884) -> (reversed array=→"Rotation signal 3":cluster{"Time":dbl[], dbl[]}[])
        n450 = case shown="Error .." w882 {
          selector: w882 -> [w891 w892]
          tunnel: [w891 w895] -> _
          frame No Error {
          }
          frame Error {
            w900 = "\r\n"
            n451 = Unbundle By Name(w892) -> ("code"=w903:i32, "source"=w901:string)
            n452 = Number To Decimal String(number=w903) -> (decimal integer string=w902:string)  [unwired: 1 in]
            n453 = Concatenate Strings("There is an error:" ("string"), w900, w902, w900, w901, w900, "Do you want to clear it?" ("string")) -> (w896:string)
            n454 = Two Button Dialog(message=w896, 1:"No" ("F button name (\"Cancel\")"), 2:"Yes" ("T button name (\"OK\")")) -> (T button?=w894:bool)
            n455 = call <vilib>:"Clear Errors.vi"("error in (no error)"=w892) -> ("error out"=w893:errorcluster)  [unwired: 5 in, 1 out]
            n456 = Select(t=w893, s=w894, f=w892) -> (s? t:f=w895:errorcluster)
          }
        }
      }
      event "AOC": Mouse Down {
        n457 = event-data() -> ()  [unwired: 1 in, 8 out]
        n458 = Look In Map(map=w985, key="pulse Y") -> (value=w1000:i32)  [unwired: 1 in, 1 out]
        n459 = Look In Map(map=w983, key="Y pi/2") -> (value=w998:dbl)  [unwired: 1 in, 1 out]
        n460 = Look In Map(map=w983, key="Delay") -> (value=w997:dbl)  [unwired: 1 in, 1 out]
        n461 = Look In Map(map=w985, key="pulse Z") -> (value=w994:i32)  [unwired: 1 in, 1 out]
        n462 = Look In Map(map=w983, key="Z pi/4") -> (value=w991:dbl)  [unwired: 1 in, 1 out]
        n463 = Look In Map(map=w983, key="Delay") -> (value=w992:dbl)  [unwired: 1 in, 1 out]
        n464 = call "Add_to_sequence_SubVI_v1.vi"("Delay [us]"=w997, "Pulse length [us]"=w998, "Channel number"=w1000, "Array sequence in"=w1001) -> ("Array sequence out"=w996:cluster{"Timing 0":dbl[]}[])
        n465 = call "Add_to_sequence_SubVI_v1.vi"("Delay [us]"=w992, "Pulse length [us]"=w991, "Channel number"=w994, "Array sequence in"=w996) -> ("Array sequence out"=w986:cluster{"Timing 0":dbl[]}[])
        n466 = Wait (ms)(milliseconds to wait=u32 150) -> ()  [unwired: 1 out]
        n467 = Look In Map(map=w985, key="pulse Y") -> (value=w981:i32)  [unwired: 1 in, 1 out]
        n468 = Look In Map(map=w983, key="Y pi/2") -> (value=w980:dbl)  [unwired: 1 in, 1 out]
        n469 = Look In Map(map=w983, key="Delay") -> (value=w979:dbl)  [unwired: 1 in, 1 out]
        n470 = call "Add_to_sequence_SubVI_v1.vi"("Delay [us]"=w979, "Pulse length [us]"=w980, "Channel number"=w981, "Array sequence in"=w986) -> ("Array sequence out"=w978:cluster{"Timing 0":dbl[]}[])
      }
      event "X pi": Mouse Down {
        n471 = event-data() -> ()  [unwired: 1 in, 8 out]
        n472 = Look In Map(map=w1007, key="X pi") -> (value=w1003:dbl)  [unwired: 1 in, 1 out]
        n473 = Look In Map(map=w1007, key="Delay") -> (value=w1002:dbl)  [unwired: 1 in, 1 out]
        n474 = Look In Map(map=w1013, key="pulse X") -> (value=w1004:i32)  [unwired: 1 in, 1 out]
        n475 = Wait (ms)(milliseconds to wait=u32 150) -> ()  [unwired: 1 out]
        n476 = call "Add_to_sequence_SubVI_v1.vi"("Delay [us]"=w1002, "Pulse length [us]"=w1003, "Channel number"=w1004, "Array sequence in"=w1006) -> ("Array sequence out"=w1005:cluster{"Timing 0":dbl[]}[])
      }
      event "X pi/2": Mouse Down {
        n477 = event-data() -> ()  [unwired: 1 in, 8 out]
        n478 = Look In Map(map=w1019, key="X pi/2") -> (value=w1015:dbl)  [unwired: 1 in, 1 out]
        n479 = Look In Map(map=w1019, key="Delay") -> (value=w1014:dbl)  [unwired: 1 in, 1 out]
        n480 = Look In Map(map=w1025, key="pulse X") -> (value=w1016:i32)  [unwired: 1 in, 1 out]
        n481 = Wait (ms)(milliseconds to wait=u32 150) -> ()  [unwired: 1 out]
        n482 = call "Add_to_sequence_SubVI_v1.vi"("Delay [us]"=w1014, "Pulse length [us]"=w1015, "Channel number"=w1016, "Array sequence in"=w1018) -> ("Array sequence out"=w1017:cluster{"Timing 0":dbl[]}[])
      }
      event "X pi/4": Mouse Down {
        n483 = event-data() -> ()  [unwired: 1 in, 8 out]
        n484 = Look In Map(map=w1036, key="pulse X") -> (value=w1032:i32)  [unwired: 1 in, 1 out]
        n485 = Look In Map(map=w1034, key="X pi/4") -> (value=w1031:dbl)  [unwired: 1 in, 1 out]
        n486 = Look In Map(map=w1034, key="Delay") -> (value=w1030:dbl)  [unwired: 1 in, 1 out]
        n487 = Wait (ms)(milliseconds to wait=u32 150) -> ()  [unwired: 1 out]
        n488 = call "Add_to_sequence_SubVI_v1.vi"("Delay [us]"=w1030, "Pulse length [us]"=w1031, "Channel number"=w1032, "Array sequence in"=w1029) -> ("Array sequence out"=w1028:cluster{"Timing 0":dbl[]}[])
      }
      event "Y pi": Mouse Down {
        n489 = event-data() -> ()  [unwired: 1 in, 8 out]
        n490 = Look In Map(map=w1042, key="Y pi") -> (value=w1038:dbl)  [unwired: 1 in, 1 out]
        n491 = Look In Map(map=w1042, key="Delay") -> (value=w1037:dbl)  [unwired: 1 in, 1 out]
        n492 = Look In Map(map=w1048, key="pulse Y") -> (value=w1039:i32)  [unwired: 1 in, 1 out]
        n493 = Wait (ms)(milliseconds to wait=u32 150) -> ()  [unwired: 1 out]
        n494 = call "Add_to_sequence_SubVI_v1.vi"("Delay [us]"=w1037, "Pulse length [us]"=w1038, "Channel number"=w1039, "Array sequence in"=w1041) -> ("Array sequence out"=w1040:cluster{"Timing 0":dbl[]}[])
      }
      event "Y pi/2": Mouse Down {
        n495 = event-data() -> ()  [unwired: 1 in, 8 out]
        n496 = Look In Map(map=w1054, key="Y pi/2") -> (value=w1050:dbl)  [unwired: 1 in, 1 out]
        n497 = Look In Map(map=w1054, key="Delay") -> (value=w1049:dbl)  [unwired: 1 in, 1 out]
        n498 = Look In Map(map=w1060, key="pulse Y") -> (value=w1051:i32)  [unwired: 1 in, 1 out]
        n499 = Wait (ms)(milliseconds to wait=u32 150) -> ()  [unwired: 1 out]
        n500 = call "Add_to_sequence_SubVI_v1.vi"("Delay [us]"=w1049, "Pulse length [us]"=w1050, "Channel number"=w1051, "Array sequence in"=w1053) -> ("Array sequence out"=w1052:cluster{"Timing 0":dbl[]}[])
      }
      event "Y pi/4": Mouse Down {
        n501 = event-data() -> ()  [unwired: 1 in, 8 out]
        n502 = Look In Map(map=w1066, key="Y pi/4") -> (value=w1062:dbl)  [unwired: 1 in, 1 out]
        n503 = Look In Map(map=w1066, key="Delay") -> (value=w1061:dbl)  [unwired: 1 in, 1 out]
        n504 = Look In Map(map=w1072, key="pulse Y") -> (value=w1063:i32)  [unwired: 1 in, 1 out]
        n505 = Wait (ms)(milliseconds to wait=u32 150) -> ()  [unwired: 1 out]
        n506 = call "Add_to_sequence_SubVI_v1.vi"("Delay [us]"=w1061, "Pulse length [us]"=w1062, "Channel number"=w1063, "Array sequence in"=w1065) -> ("Array sequence out"=w1064:cluster{"Timing 0":dbl[]}[])
      }
      event "Z pi": Mouse Down {
        n507 = event-data() -> ()  [unwired: 1 in, 8 out]
        n508 = Look In Map(map=w1078, key="Z pi") -> (value=w1074:dbl)  [unwired: 1 in, 1 out]
        n509 = Look In Map(map=w1078, key="Delay") -> (value=w1073:dbl)  [unwired: 1 in, 1 out]
        n510 = Look In Map(map=w1084, key="pulse Z") -> (value=w1075:i32)  [unwired: 1 in, 1 out]
        n511 = Wait (ms)(milliseconds to wait=u32 150) -> ()  [unwired: 1 out]
        n512 = call "Add_to_sequence_SubVI_v1.vi"("Delay [us]"=w1073, "Pulse length [us]"=w1074, "Channel number"=w1075, "Array sequence in"=w1077) -> ("Array sequence out"=w1076:cluster{"Timing 0":dbl[]}[])
      }
      event "Z pi/2": Mouse Down {
        n513 = event-data() -> ()  [unwired: 1 in, 8 out]
        n514 = Look In Map(map=w1090, key="Z pi/2") -> (value=w1086:dbl)  [unwired: 1 in, 1 out]
        n515 = Look In Map(map=w1090, key="Delay") -> (value=w1085:dbl)  [unwired: 1 in, 1 out]
        n516 = Look In Map(map=w1096, key="pulse Z") -> (value=w1087:i32)  [unwired: 1 in, 1 out]
        n517 = Wait (ms)(milliseconds to wait=u32 150) -> ()  [unwired: 1 out]
        n518 = call "Add_to_sequence_SubVI_v1.vi"("Delay [us]"=w1085, "Pulse length [us]"=w1086, "Channel number"=w1087, "Array sequence in"=w1089) -> ("Array sequence out"=w1088:cluster{"Timing 0":dbl[]}[])
      }
      event "Z pi/4": Mouse Down {
        n519 = event-data() -> ()  [unwired: 1 in, 8 out]
        n520 = Look In Map(map=w1102, key="Z pi/4") -> (value=w1098:dbl)  [unwired: 1 in, 1 out]
        n521 = Look In Map(map=w1102, key="Delay") -> (value=w1097:dbl)  [unwired: 1 in, 1 out]
        n522 = Look In Map(map=w1108, key="pulse Z") -> (value=w1099:i32)  [unwired: 1 in, 1 out]
        n523 = Wait (ms)(milliseconds to wait=u32 150) -> ()  [unwired: 1 out]
        n524 = call "Add_to_sequence_SubVI_v1.vi"("Delay [us]"=w1097, "Pulse length [us]"=w1098, "Channel number"=w1099, "Array sequence in"=w1101) -> ("Array sequence out"=w1100:cluster{"Timing 0":dbl[]}[])
      }
      event "Add pulse": Mouse Down {
        # "If it is nonlinear coil, it should be waited for much more time.\nBecause the pulse shape of the nonlinear coil is not good. It still affects the atom  after the pulse pauses"
        # "The nonlinear coil value"
        n525 = event-data() -> ()  [unwired: 1 in, 8 out]
        n526 = property on="Channel" class="Ring (strict)"() -> ("Value"=w1110:u16)  [unwired: 2 in, 2 out]
        n527 = Equal?(x=w1110, y=u16 9) -> (x = y?=w1112:bool)
        n528 = Index Array(array=w1113, index="Channel") -> (element=w1121:string)
        n529 = Look In Map(map=w1122, key=w1121) -> (value=w1111:i32)  [unwired: 1 in, 1 out]
        n530 = case shown="True" w1112 {
          tunnel: w1118 -> [w1125 w1131]
          tunnel: [w1124 w1128] -> w1115
          frame False {
            n531 = Look In Map(map=w1125, key="Delay") -> (value=w1124:dbl)  [unwired: 1 in, 1 out]
          }
          frame True {
            n532 = Look In Map(map=w1131, key="Delay") -> (value=w1129:dbl)  [unwired: 1 in, 1 out]
            n533 = Add(x=50.0, y=w1129) -> (x+y=w1128:dbl)
          }
        }
        n534 = Wait (ms)(milliseconds to wait=u32 150) -> ()  [unwired: 1 out]
        n535 = call "Add_to_sequence_SubVI_v1.vi"("Delay [us]"=w1115, "Pulse length [us]"="Time [us]", "Channel number"=w1111, "Array sequence in"=w1117) -> ("Array sequence out"=w1116:cluster{"Timing 0":dbl[]}[])
      }
      event "Add pulse advanced": Mouse Down {
        # "Search for choosen channels"
        n536 = event-data() -> ()  [unwired: 1 in, 8 out]
        n537 = for {
          tunnel: "Physical channels" -> [w1151] mode=indexing
          tunnel: w1144 -> [w1152]
          tunnel: [w1150] -> w1143 mode=indexing
          tunnel: [w1148] -> w1140 mode=indexing
          n538 = Search 1D Array(1D array=w1152, element=w1151) -> (index of element=w1150:i32)  [unwired: 1 in]
          n539 = Equal?(x=w1150, y=-1) -> (x = y?=w1148:bool)
        }
        n540 = Or Array Elements(Boolean array=w1140) -> (logical OR=w1139:bool)
        n541 = case shown="True" w1139 {
          frame False {
          }
          frame True {
            n542 = One Button Dialog(message="Some port names are not correct!!!\nPulse sequance may not be correct!") -> ()  [unwired: 1 in, 1 out]
          }
        }
        n543 = for {
          tunnel: w1146 -> [w1154] mode=indexing
          tunnel: w1143 -> [w1158]
          tunnel: [w1153] -> w1136 mode=indexing
          i -> [w1157]
          n544 = for {
            tunnel: w1158 -> [w1174] mode=indexing
            tunnel: w1157 -> [w1175]
            tunnel: [w1173] -> w1156 mode=indexing
            n545 = Equal?(x=w1174, y=w1175) -> (x = y?=w1173:bool)
          }
          n546 = Or Array Elements(Boolean array=w1156) -> (logical OR=w1155:bool)
          n547 = case shown="True" w1155 {
            tunnel: w1154 -> [w1161 w1168]
            tunnel: [w1159 w1166] -> w1153
            frame True {
              n548 = local read "Time [us]"() -> (w1160:dbl)
              n549 = in-place {
                in-place-border: w1160 -> [w1164]
                n550 = in-place-cluster #9(w1161) -> ("Timing 0"=w1165:dbl[])
                n551 = Build Array (concatenate)(w1165, w1164, 0.0 ("element")) -> (w1162:dbl[])
                n552 = in-place-cluster #9("Timing 0"=w1162) -> (w1159:cluster{"Timing 0":dbl[]})
              }
            }
            frame False {
              n553 = local read "Time [us]"() -> (w1167:dbl)
              n554 = in-place {
                in-place-border: w1167 -> [w1170]
                n555 = in-place-cluster #10(w1168) -> ("Timing 0"=w1172:dbl[])
                n556 = Build Array (concatenate)(w1172, 0.0 ("element"), w1170) -> (w1171:dbl[])
                n557 = in-place-cluster #10("Timing 0"=w1171) -> (w1166:cluster{"Timing 0":dbl[]})
              }
            }
          }
        }
        n558 = Look In Map(map=w1138, key="Delay") -> (value=w1132:dbl)  [unwired: 1 in, 1 out]
        n559 = Wait (ms)(milliseconds to wait=u32 150) -> ()  [unwired: 1 out]
        n560 = call "Add_to_sequence_SubVI_v1.vi"("Delay [us]"=w1132, "Pulse length [us]"=0.0, "Channel number"=-1, "Array sequence in"=w1136) -> ("Array sequence out"=w1135:cluster{"Timing 0":dbl[]}[])
      }
      event "Save single sequence": Mouse Down {
        n561 = event-data() -> ()  [unwired: 1 in, 8 out]
        n562 = Look In Map(map=w1198, key="Accqusition TRIG") -> (value=w1188:i32)  [unwired: 1 in, 1 out]
        n563 = Look In Map(map=w1195, key="TTL") -> (value=w1187:dbl)  [unwired: 1 in, 1 out]
        n564 = Look In Map(map=w1195, key="Delay") -> (value=w1186:dbl)  [unwired: 1 in, 1 out]
        n565 = Look In Map(map=w1195, key="Probe") -> (value=w1190:dbl)  [unwired: 1 in, 1 out]
        n566 = for {
          tunnel: w1185 -> [w1207] mode=indexing
          tunnel: w1187 -> [w1206]
          tunnel: [w1205] -> w1189 mode=indexing
          tunnel: w1188 -> [w1204]
          i -> [w1203]
          n567 = Equal?(x=w1204, y=w1203) -> (x = y?=w1208:bool)
          n568 = case shown="True" w1208 {
            tunnel: w1207 -> [w1209 w1212]
            tunnel: w1206 -> [_ w1211]
            tunnel: [w1209 w1210] -> w1205
            frame False {
            }
            frame True {
              n569 = in-place {
                in-place-border: w1211 -> [w1213]
                n570 = in-place-cluster #11(w1212) -> ("Timing 0"=w1214:dbl[])
                n571 = Build Array (concatenate)(w1214, w1213) -> (w1215:dbl[])
                n572 = in-place-cluster #11("Timing 0"=w1215) -> (w1210:cluster{"Timing 0":dbl[]})
              }
            }
          }
        }
        n573 = Look In Map(map=w1198, key="Keithley TRIG") -> (value=w1193:i32)  [unwired: 1 in, 1 out]
        n574 = for {
          tunnel: w1189 -> [w1236] mode=indexing
          tunnel: w1193 -> [w1238]
          tunnel: w1187 -> [w1235]
          tunnel: w1186 -> [w1234]
          tunnel: [w1233] -> w1191 mode=indexing
          i -> [w1239]
          n575 = Equal?(x=w1239, y=w1238) -> (x = y?=w1237:bool)
          n576 = case shown="True" w1237 {
            tunnel: w1236 -> [w1240 w1244]
            tunnel: w1235 -> [_ w1243]
            tunnel: w1234 -> [_ w1242]
            tunnel: [w1240 w1241] -> w1233
            frame False {
            }
            frame True {
              n577 = in-place {
                in-place-border: w1243 -> [w1248]
                in-place-border: w1242 -> [w1247]
                n578 = in-place-cluster #12(w1244) -> ("Timing 0"=w1250:dbl[])
                n579 = Multiply(x=2.0, y=w1247) -> (x*y=w1245:dbl)
                n580 = Build Array (concatenate)(w1250, 0.0, w1245, w1248) -> (w1251:dbl[])
                n581 = in-place-cluster #12("Timing 0"=w1251) -> (w1241:cluster{"Timing 0":dbl[]})
              }
            }
          }
        }
        n582 = Look In Map(map=w1198, key="LD probe") -> (value=w1192:i32)  [unwired: 1 in, 1 out]
        n583 = flat-sequence {
          frame #0 {
            n584 = Wait (ms)(milliseconds to wait=u32 150) -> ()  [unwired: 1 out]
          }
          frame #1 {
            n585 = invoke on="Save single sequence" class="Bool (strict)" method="Reinit To Default"() -> ()  [unwired: 3 in, 3 out]
          }
        }
        n586 = for {
          tunnel: w1192 -> [w1221]
          tunnel: w1191 -> [w1219] mode=indexing
          tunnel: w1190 -> [w1218]
          tunnel: [w1217] -> w1184 mode=indexing
          tunnel: w1186 -> [w1216]
          i -> [w1222]
          n587 = Equal?(x=w1222, y=w1221) -> (x = y?=w1220:bool)
          n588 = case shown="True" w1220 {
            tunnel: w1219 -> [w1223 w1227]
            tunnel: [w1223 w1226] -> w1217
            tunnel: w1218 -> [_ w1225]
            tunnel: w1216 -> [_ w1224]
            frame False {
            }
            frame True {
              n589 = in-place {
                in-place-border: w1225 -> [w1228]
                in-place-border: w1224 -> [w1229]
                n590 = in-place-cluster #13(w1227) -> ("Timing 0"=w1231:dbl[])
                n591 = Build Array (concatenate)(w1231, 0.0, w1229, w1228) -> (w1232:dbl[])
                n592 = in-place-cluster #13("Timing 0"=w1232) -> (w1226:cluster{"Timing 0":dbl[]})
              }
            }
          }
        }
        n593 = call "Array_to_cluster_sequence_SubVI_v1.vi"("Array"=w1184) -> ("Sequence"=w1183:T6)
        n594 = local read "Sampling data"() -> (w1181:T2)
        n595 = local read "Config folder"() -> (w1178:string)
        n596 = Concatenate Strings(w1178, "\\pulse_sequence_DAQ.ini" ("string")) -> (w1176:string)
        n597 = call "Set_Pulse_Seq_DAQ.vi"("Time Unit"=T12 {"Time Unit"=enum."MicroSecond"}, "error in"=w1180, "Sampling data"=w1181, "Sequence"=w1183, "Filename (ini)"=w1176) -> ("error out"=w1179:errorcluster)  [unwired: 6 in]
      }
      event "Save multi Sequence": Mouse Down {
        n598 = event-data() -> ()  [unwired: 1 in, 8 out]
        n599 = local read "Config folder"() -> (w1253:string)
        n600 = call <vilib>:"Application Directory.vi"() -> ("Application Directory"=w1262:path)
        n601 = Concatenate Strings(w1253, "\\temp_multi_FID\\" ("string")) -> (w1252:string)
        n602 = Concatenate Strings("Config_Files\\" ("string"), w1252) -> (w1259:string)
        n603 = String To Path(string=w1259) -> (path=w1261:path)
        n604 = Build Path(base path=w1262, name or relative path=w1261) -> (appended path=w1260:path)
        n605 = call <userlib>:"List Directory__ogtk.vi"("directory path"=w1260) -> ("file names"=w1258:string[])  [unwired: 3 in, 3 out]
        n606 = for {
          tunnel: w1258 -> [w1270] mode=indexing
          shift-right: [w1271] -> w1257
          shift-left: w1256 -> [w1272]
          tunnel: w1252 -> [w1269]
          n607 = Concatenate Strings(w1269, w1270) -> (w1273:string)
          n608 = call "Delete_file.vi"("error in"=w1272, "Filename (ini)"=w1273) -> ("error out"=w1271:errorcluster)  [unwired: 9 in]
        }
        n609 = for {
          N: "Period number" -> [_]
          tunnel: w1268 -> [w1280]
          tunnel: w1267 -> [w1277]
          tunnel: w1266 -> [w1286]
          tunnel: "Period [us]" -> [w1303]
          tunnel: w1257 -> [w1294]
          tunnel: [w1292] -> w1263
          i -> [w1288]
          # "Write the full number in the name to store the data\n 1-->001\n10-->010\n100-->100"
          n610 = Multiply(x=w1303, y=w1288) -> (x*y=w1284:dbl)
          n611 = Look In Map(map=w1280, key="Nonlinear coil") -> (value=w1285:i32)  [unwired: 1 in, 1 out]
          n612 = Look In Map(map=w1277, key="Delay") -> (value=w1283:dbl)  [unwired: 1 in, 1 out]
          n613 = Look In Map(map=w1280, key="pulse X") -> (value=w1278:i32)  [unwired: 1 in, 1 out]
          n614 = call "Add_to_sequence_SubVI_Directly.vi"("Delay [us]"=w1283, "Pulse length [us]"=w1284, "Channel number"=w1285, "Array sequence in"=w1286) -> ("Array sequence out"=w1282:cluster{"Timing 0":dbl[]}[])
          n615 = Look In Map(map=w1277, key="TTL") -> (value=w1304:dbl)  [unwired: 1 in, 1 out]
          n616 = Look In Map(map=w1277, key="Delay") -> (value=w1274:dbl)  [unwired: 1 in, 1 out]
          n617 = Look In Map(map=w1277, key="Probe") -> (value=w1307:dbl)  [unwired: 1 in, 1 out]
          n618 = Look In Map(map=w1277, key="X pi/4") -> (value=w1275:dbl)  [unwired: 1 in, 1 out]
          n619 = call "Add_to_sequence_SubVI_v1.vi"("Delay [us]"=w1274, "Pulse length [us]"=w1275, "Channel number"=w1278, "Array sequence in"=w1282) -> ("Array sequence out"=w1281:cluster{"Timing 0":dbl[]}[])
          n620 = Look In Map(map=w1280, key="Accqusition TRIG") -> (value=w1305:i32)  [unwired: 1 in, 1 out]
          n621 = for {
            tunnel: w1281 -> [w1337] mode=indexing
            tunnel: w1304 -> [w1336]
            tunnel: [w1335] -> w1306 mode=indexing
            tunnel: w1305 -> [w1334]
            i -> [w1333]
            n622 = Equal?(x=w1334, y=w1333) -> (x = y?=w1338:bool)
            n623 = case shown="True" w1338 {
              tunnel: w1337 -> [w1339 w1342]
              tunnel: w1336 -> [_ w1341]
              tunnel: [w1339 w1340] -> w1335
              frame False {
              }
              frame True {
                n624 = in-place {
                  in-place-border: w1341 -> [w1343]
                  n625 = in-place-cluster #14(w1342) -> ("Timing 0"=w1344:dbl[])
                  n626 = Build Array (concatenate)(w1344, w1343) -> (w1345:dbl[])
                  n627 = in-place-cluster #14("Timing 0"=w1345) -> (w1340:cluster{"Timing 0":dbl[]})
                }
              }
            }
          }
          n628 = Look In Map(map=w1280, key="Keithley TRIG") -> (value=w1310:i32)  [unwired: 1 in, 1 out]
          n629 = for {
            tunnel: w1306 -> [w1366] mode=indexing
            tunnel: w1310 -> [w1368]
            tunnel: w1304 -> [w1365]
            tunnel: w1274 -> [w1364]
            tunnel: [w1363] -> w1308 mode=indexing
            i -> [w1369]
            n630 = Equal?(x=w1369, y=w1368) -> (x = y?=w1367:bool)
            n631 = case shown="True" w1367 {
              tunnel: w1366 -> [w1370 w1374]
              tunnel: w1365 -> [_ w1373]
              tunnel: w1364 -> [_ w1372]
              tunnel: [w1370 w1371] -> w1363
              frame False {
              }
              frame True {
                n632 = in-place {
                  in-place-border: w1373 -> [w1378]
                  in-place-border: w1372 -> [w1377]
                  n633 = in-place-cluster #15(w1374) -> ("Timing 0"=w1380:dbl[])
                  n634 = Multiply(x=2.0, y=w1377) -> (x*y=w1375:dbl)
                  n635 = Build Array (concatenate)(w1380, 0.0, w1375, w1378) -> (w1381:dbl[])
                  n636 = in-place-cluster #15("Timing 0"=w1381) -> (w1371:cluster{"Timing 0":dbl[]})
                }
              }
            }
          }
          n637 = Look In Map(map=w1280, key="LD probe") -> (value=w1309:i32)  [unwired: 1 in, 1 out]
          n638 = for {
            tunnel: w1309 -> [w1351]
            tunnel: w1308 -> [w1349] mode=indexing
            tunnel: w1307 -> [w1348]
            tunnel: [w1347] -> w1300 mode=indexing
            tunnel: w1274 -> [w1346]
            i -> [w1352]
            n639 = Equal?(x=w1352, y=w1351) -> (x = y?=w1350:bool)
            n640 = case shown="True" w1350 {
              tunnel: w1349 -> [w1353 w1357]
              tunnel: [w1353 w1356] -> w1347
              tunnel: w1348 -> [_ w1355]
              tunnel: w1346 -> [_ w1354]
              frame False {
              }
              frame True {
                n641 = in-place {
                  in-place-border: w1355 -> [w1358]
                  in-place-border: w1354 -> [w1359]
                  n642 = in-place-cluster #16(w1357) -> ("Timing 0"=w1361:dbl[])
                  n643 = Build Array (concatenate)(w1361, 0.0, w1359, w1358) -> (w1362:dbl[])
                  n644 = in-place-cluster #16("Timing 0"=w1362) -> (w1356:cluster{"Timing 0":dbl[]})
                }
              }
            }
          }
          n645 = Less?(x=w1288, y=10) -> (x < y?=w1289:bool)
          n646 = case shown="False" w1289 {
            tunnel: [w1317 w1328] -> w1287
            tunnel: w1288 -> [w1318 w1331]
            frame False {
              n647 = Less?(x=w1318, y=100) -> (x < y?=w1319:bool)
              n648 = case shown="False" w1319 {
                tunnel: w1318 -> [w1322 w1326]
                tunnel: [w1321 w1323] -> w1317
                frame False {
                  (unwired) i16 1 ("width (-)")
                  n649 = Number To Decimal String(number=w1322) -> (decimal integer string=w1321:string)  [unwired: 1 in]
                }
                frame True {
                  n650 = Number To Decimal String(number=w1326, width (-)=i16 1) -> (decimal integer string=w1325:string)
                  n651 = Concatenate Strings("0" ("string"), w1325) -> (w1323:string)
                }
              }
            }
            frame True {
              n652 = Number To Decimal String(number=w1331, width (-)=i16 1) -> (decimal integer string=w1330:string)
              n653 = Concatenate Strings("00" ("string"), w1330) -> (w1328:string)
            }
          }
          n654 = call "Array_to_cluster_sequence_SubVI_v1.vi"("Array"=w1300) -> ("Sequence"=w1293:T6)
          n655 = local read "Sampling data"() -> (w1297:T2)
          n656 = local read "Config folder"() -> (w1298:string)
          n657 = Concatenate Strings(w1298, "\\temp_multi_FID\\Single_FID_" ("string"), w1287, ".ini" ("string")) -> (w1299:string)
          n658 = call "Set_Pulse_Seq_DAQ.vi"("Time Unit"=T12 {"Time Unit"=enum."MicroSecond"}, "error in"=w1294, "Sampling data"=w1297, "Sequence"=w1293, "Filename (ini)"=w1299) -> ("error out"=w1292:errorcluster)  [unwired: 6 in]
        }
        n659 = flat-sequence {
          frame #0 {
            n660 = Wait (ms)(milliseconds to wait=u32 150) -> ()  [unwired: 1 out]
          }
          frame #1 {
            n661 = invoke on="Save single sequence" class="Bool (strict)" method="Reinit To Default"() -> ()  [unwired: 3 in, 3 out]
          }
        }
      }
      event "Save for tomography": Mouse Down {
        w1389 = string[][] [["None", "None"], ["Y pi", "None"], ["Z pi/2", "Y pi"]]
        w1383 = string[] ["None", "Y pi/2", "X pi/2"]
        # "Additional delay to ensure that\nall measurement start at the\nsame moment"
        # "CYCLOPS"
        # "Control pulses"
        n662 = event-data() -> ()  [unwired: 1 in, 8 out]
        n663 = local write "pulses type (priv)"(w1383) -> ()
        n664 = for {
          tunnel: w1391 -> [w1519]
          tunnel: w1383 -> [w1518] mode=indexing
          tunnel: [w1517] -> w1398 mode=indexing
          # "Check longest control pulse"
          n665 = Look In Map(map=w1519, key=w1518) -> (value=w1517:dbl)  [unwired: 1 in, 1 out]
        }
        n666 = Look In Map(map=w1391, key="Delay") -> (value=w1396:dbl)  [unwired: 1 in, 1 out]
        n667 = for {
          tunnel: w1391 -> [w1525]
          tunnel: w1389 -> [w1524] mode=indexing
          tunnel: w1396 -> [w1521]
          tunnel: [w1520] -> w1397 mode=indexing
          # "Check longest CYCLOPS sequence"
          n668 = for {
            tunnel: w1525 -> [w1528]
            tunnel: [w1527] -> w1523 mode=indexing
            tunnel: w1524 -> [w1526] mode=indexing
            n669 = Look In Map(map=w1528, key=w1526) -> (value=w1527:dbl)  [unwired: 1 in, 1 out]
          }
          n670 = Add Array Elements(numeric array=w1523) -> (sum=w1522:dbl)
          n671 = Add(x=w1522, y=w1521) -> (x+y=w1520:dbl)
        }
        n672 = for {
          tunnel: w1398 -> [w1515] mode=indexing
          tunnel: w1397 -> [w1516]
          tunnel: w1396 -> [w1513]
          tunnel: [w1514] -> w1394 mode=indexing
          n673 = Compound Arithmetic op=unknown(w1516, w1513, w1515, w1513) -> (w1514:dbl[])
        }
        n674 = Array Max & Min(array=w1394) -> (max value=w1395:dbl)  [unwired: 3 out]
        n675 = Subtract(x=w1395, y=w1394) -> (x-y=w1388:dbl[][])
        n676 = for {
          tunnel: string[] ["None", "pulse Y", "pulse X"] -> [w1425] mode=indexing
          tunnel: w1383 -> [w1426] mode=indexing
          tunnel: w1387 -> [w1427]
          tunnel: w1392 -> [w1416]
          tunnel: w1391 -> [w1417]
          tunnel: string[][] [["None", "None"], ["pulse Y", "None"], ["pulse Z", "pulse Y"]] -> [w1420]
          tunnel: w1389 -> [w1419]
          tunnel: [w1415] -> w1386 mode=concatenating
          tunnel: w1388 -> [w1414] mode=indexing
          # "Iterate over control pulses"
          n677 = Look In Map(map=w1416, key=w1425) -> (value=w1423:i32)  [unwired: 1 in, 1 out]
          n678 = Look In Map(map=w1417, key=w1426) -> (value=w1422:dbl)  [unwired: 1 in, 1 out]
          n679 = Look In Map(map=w1417, key="Delay") -> (value=w1418:dbl)  [unwired: 1 in, 1 out]
          n680 = call "Add_to_sequence_SubVI_v1.vi"("Delay [us]"=w1418, "Pulse length [us]"=w1422, "Channel number"=w1423, "Array sequence in"=w1427) -> ("Array sequence out"=w1421:cluster{"Timing 0":dbl[]}[])
          n681 = for {
            tunnel: w1421 -> [w1454]
            tunnel: w1420 -> [w1451] mode=indexing
            tunnel: w1419 -> [w1452] mode=indexing
            tunnel: w1418 -> [w1453]
            tunnel: w1417 -> [w1436]
            tunnel: w1416 -> [w1432]
            tunnel: [w1435] -> w1415 mode=indexing
            tunnel: w1414 -> [w1430] mode=indexing
            # "Add equalization of the time interval"
            # "Iterate over CYCLOPS in 2 for loops because CYCLOPS consists of a few pulses"
            n682 = for {
              shift-right: [w1505] -> w1434
              shift-left: w1454 -> [w1508]
              tunnel: w1453 -> [w1504]
              tunnel: w1452 -> [w1511] mode=indexing
              tunnel: w1451 -> [w1512] mode=indexing
              tunnel: w1436 -> [w1510]
              tunnel: w1432 -> [w1509]
              tunnel: [w1504] -> w1429
              n683 = Look In Map(map=w1509, key=w1512) -> (value=w1507:i32)  [unwired: 1 in, 1 out]
              n684 = Look In Map(map=w1510, key=w1511) -> (value=w1506:dbl)  [unwired: 1 in, 1 out]
              n685 = call "Add_to_sequence_SubVI_v1.vi"("Delay [us]"=w1504, "Pulse length [us]"=w1506, "Channel number"=w1507, "Array sequence in"=w1508) -> ("Array sequence out"=w1505:cluster{"Timing 0":dbl[]}[])
            }
            n686 = Look In Map(map=w1432, key="None") -> (value=w1431:i32)  [unwired: 1 in, 1 out]
            n687 = call "Add_to_sequence_SubVI_v1.vi"("Delay [us]"=w1429, "Pulse length [us]"=w1430, "Channel number"=w1431, "Array sequence in"=w1434) -> ("Array sequence out"=w1428:cluster{"Timing 0":dbl[]}[])
            n688 = Look In Map(map=w1436, key="Probe") -> (value=w1446:dbl)  [unwired: 1 in, 1 out]
            n689 = Look In Map(map=w1436, key="Delay") -> (value=w1450:dbl)  [unwired: 1 in, 1 out]
            n690 = Look In Map(map=w1432, key="Accqusition TRIG") -> (value=w1448:i32)  [unwired: 1 in, 1 out]
            n691 = Look In Map(map=w1436, key="TTL") -> (value=w1449:dbl)  [unwired: 1 in, 1 out]
            n692 = for {
              tunnel: w1428 -> [w1459] mode=indexing
              tunnel: w1449 -> [w1458]
              tunnel: [w1457] -> w1447 mode=indexing
              tunnel: w1448 -> [w1456]
              i -> [w1455]
              n693 = Equal?(x=w1456, y=w1455) -> (x = y?=w1460:bool)
              n694 = case shown="True" w1460 {
                tunnel: w1459 -> [w1461 w1464]
                tunnel: w1458 -> [_ w1463]
                tunnel: [w1461 w1462] -> w1457
                frame False {
                }
                frame True {
                  n695 = in-place {
                    in-place-border: w1463 -> [w1465]
                    n696 = in-place-cluster #17(w1464) -> ("Timing 0"=w1466:dbl[])
                    n697 = Build Array (concatenate)(w1466, w1465) -> (w1467:dbl[])
                    n698 = in-place-cluster #17("Timing 0"=w1467) -> (w1462:cluster{"Timing 0":dbl[]})
                  }
                }
              }
            }
            n699 = Look In Map(map=w1432, key="Keithley TRIG") -> (value=w1443:i32)  [unwired: 1 in, 1 out]
            n700 = for {
              tunnel: w1447 -> [w1488] mode=indexing
              tunnel: w1443 -> [w1490]
              tunnel: w1449 -> [w1487]
              tunnel: w1450 -> [w1486]
              tunnel: [w1485] -> w1445 mode=indexing
              i -> [w1491]
              n701 = Equal?(x=w1491, y=w1490) -> (x = y?=w1489:bool)
              n702 = case shown="True" w1489 {
                tunnel: w1488 -> [w1492 w1496]
                tunnel: w1487 -> [_ w1495]
                tunnel: w1486 -> [_ w1494]
                tunnel: [w1492 w1493] -> w1485
                frame False {
                }
                frame True {
                  n703 = in-place {
                    in-place-border: w1495 -> [w1500]
                    in-place-border: w1494 -> [w1499]
                    n704 = in-place-cluster #18(w1496) -> ("Timing 0"=w1502:dbl[])
                    n705 = Multiply(x=2.0, y=w1499) -> (x*y=w1497:dbl)
                    n706 = Build Array (concatenate)(w1502, 0.0, w1497, w1500) -> (w1503:dbl[])
                    n707 = in-place-cluster #18("Timing 0"=w1503) -> (w1493:cluster{"Timing 0":dbl[]})
                  }
                }
              }
            }
            n708 = Look In Map(map=w1432, key="LD probe") -> (value=w1444:i32)  [unwired: 1 in, 1 out]
            n709 = for {
              tunnel: w1444 -> [w1473]
              tunnel: w1445 -> [w1471] mode=indexing
              tunnel: w1446 -> [w1470]
              tunnel: [w1469] -> w1435 mode=indexing
              tunnel: w1450 -> [w1468]
              i -> [w1474]
              n710 = Equal?(x=w1474, y=w1473) -> (x = y?=w1472:bool)
              n711 = case shown="True" w1472 {
                tunnel: w1471 -> [w1475 w1479]
                tunnel: [w1475 w1478] -> w1469
                tunnel: w1470 -> [_ w1477]
                tunnel: w1468 -> [_ w1476]
                frame False {
                }
                frame True {
                  n712 = in-place {
                    in-place-border: w1477 -> [w1480]
                    in-place-border: w1476 -> [w1481]
                    n713 = in-place-cluster #19(w1479) -> ("Timing 0"=w1483:dbl[])
                    n714 = Build Array (concatenate)(w1483, 0.0, w1481, w1480) -> (w1484:dbl[])
                    n715 = in-place-cluster #19("Timing 0"=w1484) -> (w1478:cluster{"Timing 0":dbl[]})
                  }
                }
              }
            }
          }
        }
        n716 = flat-sequence {
          frame #0 {
            n717 = Wait (ms)(milliseconds to wait=u32 150) -> ()  [unwired: 1 out]
          }
          frame #1 {
            n718 = invoke on="Save for tomography" class="Bool (strict)" method="Reinit To Default"() -> ()  [unwired: 3 in, 3 out]
          }
        }
        n719 = for {
          tunnel: w1386 -> [w1413] mode=indexing
          shift-right: [w1401] -> w1384
          shift-left: w1385 -> [w1411]
          i -> [w1406]
          n720 = local read "Config folder"() -> (w1408:string)
          n721 = Number To Decimal String(number=w1406, width (-)=i16 1) -> (decimal integer string=w1404:string)
          n722 = call "Array_to_cluster_sequence_SubVI_v1.vi"("Array"=w1413) -> ("Sequence"=w1412:T6)
          n723 = local read "Sampling data"() -> (w1410:T2)
          n724 = Concatenate Strings(w1408, "\\tomography\\pulse_seq_DAQ_" ("string"), w1404, ".ini" ("string")) -> (w1402:string)
          n725 = call "Set_Pulse_Seq_DAQ.vi"("Time Unit"=T12 {"Time Unit"=enum."MicroSecond"}, "error in"=w1411, "Sampling data"=w1410, "Sequence"=w1412, "Filename (ini)"=w1402) -> ("error out"=w1401:errorcluster)  [unwired: 6 in]
        }
      }
      event "Save initial state": Mouse Down {
        n726 = event-data() -> ()  [unwired: 1 in, 8 out]
        n727 = String Length(string="Name of state (initial_state_)") -> (length=w1534:i32)
        n728 = Greater Than 0?(x=w1534) -> (x > 0?=w1533:bool)
        n729 = case shown="False" w1533 {
          tunnel: "Name of state (initial_state_)" -> [_ w1555]
          tunnel: [w1542 w1548] -> w1531
          tunnel: w1530 -> [w1541 w1549]
          tunnel: w1529 -> [w1540 w1550]
          frame False {
            # "Select a Name from the Ring to Save the initial_state in the State_library"
            n730 = property on="Name of initial_state" class="Ring (strict)"() -> ("Strings []"=w1547:string[])  [unwired: 2 in, 2 out]
            n731 = Index Array(array=w1547, index="Name of initial_state") -> (element=w1544:string)
            n732 = call "Array_to_cluster_sequence_SubVI_v1.vi"("Array"=w1540) -> ("Sequence"=w1539:T6)
            n733 = local read "Config folder"() -> (w1535:string)
            n734 = local read "Sampling data"() -> (w1538:T2)
            n735 = Concatenate Strings(w1535, "\\state_library\\" ("string"), w1544, ".ini" ("string")) -> (w1537:string)
            n736 = call "Set_Pulse_Seq_DAQ.vi"("Time Unit"=T12 {"Time Unit"=enum."MicroSecond"}, "error in"=w1541, "Sampling data"=w1538, "Sequence"=w1539, "Filename (ini)"=w1537) -> ("error out"=w1542:errorcluster)  [unwired: 6 in]
          }
          frame True {
            w1552 = "initial_state_" ("true string")
            n737 = Match True/False String(2:"" ("false string"), 3:w1552, 4:w1555) -> (0:w1553:bool, 1:w1551:string)
            n738 = case shown="True" w1553 {
              tunnel: w1552 -> [_ w1575]
              tunnel: w1551 -> [_ w1574]
              tunnel: w1550 -> [_ w1573]
              tunnel: w1549 -> [w1556 w1566]
              tunnel: [w1556 w1565] -> w1548
              frame False {
                n739 = xnode "Error Ring"() -> ("error out"=w1557:errorcluster)
                n740 = call <vilib>:"Simple Error Handler.vi"("error in (no error)"=w1557) -> ()  [unwired: 4 in, 5 out]
              }
              frame True {
                # "input the name by yourself, but name pattern should be like initial_satae_"
                n741 = Concatenate Strings(w1575, w1574) -> (w1569:string)
                n742 = call "Array_to_cluster_sequence_SubVI_v1.vi"("Array"=w1573) -> ("Sequence"=w1572:T6)
                n743 = local read "Config folder"() -> (w1563:string)
                n744 = local read "Sampling data"() -> (w1567:T2)
                n745 = Concatenate Strings(w1563, "\\state_library\\" ("string"), w1569, ".ini" ("string")) -> (w1568:string)
                n746 = call "Set_Pulse_Seq_DAQ.vi"("Time Unit"=T12 {"Time Unit"=enum."MicroSecond"}, "error in"=w1566, "Sampling data"=w1567, "Sequence"=w1572, "Filename (ini)"=w1568) -> ("error out"=w1565:errorcluster)  [unwired: 6 in]
              }
            }
          }
        }
      }
      event "Save  process": Mouse Down {
        n747 = event-data() -> ()  [unwired: 1 in, 8 out]
        n748 = String Length(string="Name of process (process_)") -> (length=w1581:i32)
        n749 = Greater Than 0?(x=w1581) -> (x > 0?=w1580:bool)
        n750 = case shown="False" w1580 {
          tunnel: "Name of process (process_)" -> [_ w1602]
          tunnel: [w1589 w1595] -> w1578
          tunnel: w1577 -> [w1588 w1596]
          tunnel: w1576 -> [w1587 w1597]
          frame False {
            # "Select a Name from the Ring to Save the process in the processes"
            n751 = property on="Name of process" class="Ring (strict)"() -> ("Strings []"=w1594:string[])  [unwired: 2 in, 2 out]
            n752 = Index Array(array=w1594, index="Name of process") -> (element=w1591:string)
            n753 = call "Array_to_cluster_sequence_SubVI_v1.vi"("Array"=w1587) -> ("Sequence"=w1586:T6)
            n754 = local read "Config folder"() -> (w1582:string)
            n755 = local read "Sampling data"() -> (w1585:T2)
            n756 = Concatenate Strings(w1582, "\\process\\processes\\" ("string"), w1591, ".ini" ("string")) -> (w1584:string)
            n757 = call "Set_Pulse_Seq_DAQ.vi"("Time Unit"=T12 {"Time Unit"=enum."MicroSecond"}, "error in"=w1588, "Sampling data"=w1585, "Sequence"=w1586, "Filename (ini)"=w1584) -> ("error out"=w1589:errorcluster)  [unwired: 6 in]
          }
          frame True {
            w1599 = "process_" ("true string")
            n758 = Match True/False String(2:"" ("false string"), 3:w1599, 4:w1602) -> (0:w1600:bool, 1:w1598:string)
            n759 = case shown="True" w1600 {
              tunnel: w1599 -> [_ w1622]
              tunnel: w1598 -> [_ w1621]
              tunnel: w1597 -> [_ w1620]
              tunnel: w1596 -> [w1603 w1613]
              tunnel: [w1603 w1612] -> w1595
              frame False {
                n760 = xnode "Error Ring"() -> ("error out"=w1604:errorcluster)
                n761 = call <vilib>:"Simple Error Handler.vi"("error in (no error)"=w1604) -> ()  [unwired: 4 in, 5 out]
              }
              frame True {
                # "input the name by yourself, but name pattern should be like process_"
                n762 = Concatenate Strings(w1622, w1621) -> (w1616:string)
                n763 = call "Array_to_cluster_sequence_SubVI_v1.vi"("Array"=w1620) -> ("Sequence"=w1619:T6)
                n764 = local read "Config folder"() -> (w1610:string)
                n765 = local read "Sampling data"() -> (w1614:T2)
                n766 = Concatenate Strings(w1610, "\\process\\processes\\" ("string"), w1616, ".ini" ("string")) -> (w1615:string)
                n767 = call "Set_Pulse_Seq_DAQ.vi"("Time Unit"=T12 {"Time Unit"=enum."MicroSecond"}, "error in"=w1613, "Sampling data"=w1614, "Sequence"=w1619, "Filename (ini)"=w1615) -> ("error out"=w1612:errorcluster)  [unwired: 6 in]
              }
            }
          }
        }
      }
      event "Save QPT": Mouse Down {
        w1636 = "\\process\\init_states_sets\\" ("string")
        # "1. Clear all files in the temp_states"
        n768 = event-data() -> ()  [unwired: 1 in, 8 out]
        n769 = local read "Config folder"() -> (w1623:string)
        n770 = Concatenate Strings(w1623, "\\process\\temp_states\\" ("string")) -> (w1624:string)
        n771 = Concatenate Strings("Config_Files\\" ("string"), w1624) -> (w1629:string)
        n772 = call <vilib>:"Application Directory.vi"() -> ("Application Directory"=w1632:path)
        n773 = String To Path(string=w1629) -> (path=w1631:path)
        n774 = Build Path(base path=w1632, name or relative path=w1631) -> (appended path=w1630:path)
        n775 = Concatenate Strings(w1623, w1636) -> (w1638:string)
        n776 = call <userlib>:"List Directory__ogtk.vi"("directory path"=w1630) -> ("file names"=w1627:string[])  [unwired: 3 in, 3 out]
        n777 = for {
          tunnel: w1627 -> [w1649] mode=indexing
          shift-right: [w1650] -> w1625
          shift-left: w1626 -> [w1651]
          tunnel: w1624 -> [w1648]
          n778 = Concatenate Strings(w1648, w1649) -> (w1652:string)
          n779 = call "Delete_file.vi"("error in"=w1651, "Filename (ini)"=w1652) -> ("error out"=w1650:errorcluster)  [unwired: 9 in]
        }
        n780 = call "Read_filename.vi"("error in"=w1625, "Filename (ini)"=w1638) -> ("error out"=w1634:errorcluster, "Strings []"=w1635:string[])  [unwired: 8 in]
        n781 = Array Size(array=w1635) -> (size(s)=w1637:i32)
        n782 = Initialize Array(0.0 ("element"), w1637) -> (w1644:dbl[])
        n783 = for {
          N: w1637 -> [_]
          shift-right: [w1724] -> w1646
          shift-left: w1634 -> [w1726]
          shift-right: [w1716] -> w1642
          shift-left: w1644 -> [w1718]
          tunnel: [w1713] -> w1643 mode=indexing
          tunnel: w1623 -> [w1711]
          tunnel: w1636 -> [w1710]
          tunnel: w1635 -> [w1709] mode=indexing
          i -> [w1717]
          # "3.Look for the longest Time Sequence from the initial_State"
          # "2.Read the initial_state data from the files"
          n784 = Concatenate Strings(w1711, w1710, w1709) -> (w1725:string)
          n785 = call "Get_Pulse_Seq_DAQ.vi"("error in"=w1726, "Filename (ini)"=w1725) -> ("error out"=w1724:errorcluster, "data"=w1723:T6)  [unwired: 8 in]
          n786 = call "Squence_to_Array_SubVI.vi"("Sequence"=w1723) -> ("Array"=w1713:cluster{"Timing 0":dbl[]}[])  [unwired: 10 in]
          n787 = Index Array(array=w1713, index=0) -> (element=w1720:cluster{"Timing 0":dbl[]})
          n788 = Unbundle(w1720) -> ("Timing 0"=w1721:dbl[])
          n789 = for {
            tunnel: w1721 -> [w1728] mode=indexing
            shift-right: [w1727] -> w1714
            shift-left: 0 -> [w1729]
            n790 = Add(x=w1728, y=w1729) -> (x+y=w1727:dbl)
          }
          n791 = local read "MaxTime"() -> (w1715:dbl)
          n792 = Max & Min(x=w1715, y=w1714) -> (max(x,y)=w1719:dbl)  [unwired: 1 out]
          n793 = Replace Array Subset(array=w1718, new element=w1714, index=w1717) -> (w1716:dbl[])
          n794 = local write "MaxTime"(w1719) -> ()
        }
        n795 = for {
          tunnel: w1643 -> [w1708] mode=indexing
          tunnel: w1642 -> [w1698] mode=indexing
          tunnel: [w1706] -> w1641 mode=indexing
          tunnel: w1640 -> [w1705]
          tunnel: w1639 -> [w1702]
          # "4. Add the delay time according to the longest Time sequence"
          n796 = local read "MaxTime"() -> (w1699:dbl)
          n797 = Subtract(x=w1699, y=w1698) -> (x-y=w1707:dbl)
          n798 = Look In Map(map=w1705, key="None") -> (value=w1703:i32)  [unwired: 1 in, 1 out]
          n799 = Look In Map(map=w1702, key="Delay") -> (value=w1700:dbl)  [unwired: 1 in, 1 out]
          n800 = call "Add_to_sequence_SubVI_v1.vi"("Delay [us]"=w1700, "Pulse length [us]"=w1707, "Channel number"=w1703, "Array sequence in"=w1708) -> ("Array sequence out"=w1706:cluster{"Timing 0":dbl[]}[])
        }
        n801 = for {
          shift-right: [w1663] -> w1647
          shift-left: w1646 -> [w1657]
          tunnel: w1641 -> [w1656] mode=indexing
          tunnel: w1640 -> [w1653]
          tunnel: w1639 -> [w1654]
          i -> [w1655]
          # "5. Detect the initial_state"
          # "6. Add the Process data to detect the output_state"
          n802 = local read "Process Array"() -> (w1659:cluster{"Timing 0":dbl[]}[])
          n803 = call "Add_Time_Seq.vi"("Process Array"=w1659, "Initial State Array"=w1656) -> ("Total Array"=w1658:cluster{"Timing 0":dbl[]}[])  [unwired: 9 in]
          n804 = call "Create_Time_Seq.vi"("pulses"=w1654, "Channels and actions"=w1653, "Array sequence in"=w1656) -> ("Array out"=w1661:cluster{"Timing 0":dbl[]}[][])  [unwired: 8 in]
          n805 = call "Create_Time_Seq.vi"("pulses"=w1654, "Channels and actions"=w1653, "Array sequence in"=w1658) -> ("Array out"=w1660:cluster{"Timing 0":dbl[]}[][])  [unwired: 8 in]
          n806 = Insert Into Array(array=w1661, new element=w1660) -> (w1662:cluster{"Timing 0":dbl[]}[][])  [unwired: 2 in]
          n807 = for {
            tunnel: w1662 -> [w1681] mode=indexing
            shift-right: [w1673] -> w1663
            shift-left: w1657 -> [w1674]
            tunnel: w1655 -> [w1668]
            i -> [w1671]
            # "Write the full number in the name to store the data\n 1-->001\n10-->010\n100-->100"
            n808 = Multiply(x=i16 18, y=w1668) -> (x*y=w1670:i32)
            n809 = Add(x=w1671, y=w1670) -> (x+y=w1666:i32)
            n810 = local read "Config folder"() -> (w1667:string)
            n811 = Less?(x=w1666, y=10) -> (x < y?=w1664:bool)
            n812 = case shown="False" w1664 {
              tunnel: [w1682 w1693] -> w1679
              tunnel: w1666 -> [w1683 w1696]
              frame False {
                n813 = Less?(x=w1683, y=100) -> (x < y?=w1684:bool)
                n814 = case shown="False" w1684 {
                  tunnel: w1683 -> [w1687 w1691]
                  tunnel: [w1686 w1688] -> w1682
                  frame False {
                    (unwired) i16 1 ("width (-)")
                    n815 = Number To Decimal String(number=w1687) -> (decimal integer string=w1686:string)  [unwired: 1 in]
                  }
                  frame True {
                    n816 = Number To Decimal String(number=w1691, width (-)=i16 1) -> (decimal integer string=w1690:string)
                    n817 = Concatenate Strings("0" ("string"), w1690) -> (w1688:string)
                  }
                }
              }
              frame True {
                n818 = Number To Decimal String(number=w1696, width (-)=i16 1) -> (decimal integer string=w1695:string)
                n819 = Concatenate Strings("00" ("string"), w1695) -> (w1693:string)
              }
            }
            n820 = call "Array_to_cluster_sequence_SubVI_v1.vi"("Array"=w1681) -> ("Sequence"=w1677:T6)
            n821 = local read "Sampling data"() -> (w1672:T2)
            n822 = Concatenate Strings(w1667, "\\process\\temp_states\\QPT_" ("string"), w1679, ".ini" ("string")) -> (w1676:string)
            n823 = call "Set_Pulse_Seq_DAQ.vi"("Time Unit"=T12 {"Time Unit"=enum."MicroSecond"}, "error in"=w1674, "Sampling data"=w1672, "Sequence"=w1677, "Filename (ini)"=w1676) -> ("error out"=w1673:errorcluster)  [unwired: 6 in]
          }
        }
      }
      event "State_update": Mouse Down; "initial_state_show": Value Change {
        w1730 = "Config_Ver_2\\state_library\\"
        n824 = event-data() -> ()  [unwired: 1 in, 4 out]
        n825 = flat-sequence {
          tunnel: w1737 -> [w1745]
          tunnel: [w1744] -> w1739
          tunnel: w1730 -> [w1743]
          tunnel: [w1740] -> w1733
          tunnel: "Config_Files\\" ("string") -> [w1741]
          tunnel: w1730 -> [w1740]
          tunnel: w1739 -> [w1753]
          tunnel: "initial_state_show" -> [w1752]
          tunnel: [w1753] -> w1735
          tunnel: [w1751] -> w1734
          tunnel: w1733 -> [w1751]
          tunnel: [w1750] -> w1732
          tunnel: [w1756] -> w1736
          tunnel: w1735 -> [w1757]
          tunnel: w1734 -> [w1761]
          tunnel: w1732 -> [w1758]
          frame #0 {
            # "Open the state_library to the show the files"
            n826 = Concatenate Strings(w1741, w1743) -> (w1742:string)
            n827 = String To Path(string=w1742) -> (path=w1748:path)
            n828 = call <vilib>:"Application Directory.vi"() -> ("Application Directory"=w1749:path)
            n829 = Build Path(base path=w1749, name or relative path=w1748) -> (appended path=w1747:path)
            n830 = call <userlib>:"List Directory__ogtk.vi"("error in (no error)"=w1745, "directory path"=w1747) -> ("error out"=w1744:errorcluster, "file names"=w1746:string[])  [unwired: 2 in, 2 out]
            n831 = property on="initial_state_show" class="Ring (strict)"("Strings []"=w1746) -> ()  [unwired: 2 in, 2 out]
          }
          frame #1 {
            # "Check the initial_states in the Library"
            n832 = property on="initial_state_show" class="Ring (strict)"() -> ("Strings []"=w1754:string[])  [unwired: 2 in, 2 out]
            n833 = Index Array(array=w1754, index=w1752) -> (element=w1750:string)
            n834 = local write "Initial_state_name"(w1750) -> ()
          }
          frame #2 {
            # "Show the Pulse_Sequence"
            n835 = String Length(string=w1758) -> (length=w1760:i32)
            n836 = Concatenate Strings(w1761, w1758) -> (w1755:string)
            n837 = Greater Than 0?(x=w1760) -> (x > 0?=w1759:bool)
            n838 = case shown="True" w1759 {
              tunnel: w1755 -> [_ w1768]
              tunnel: w1757 -> [w1762 w1765]
              tunnel: [w1762 w1764] -> w1756
              frame False {
              }
              frame True {
                n839 = call "Get_Pulse_Seq_DAQ.vi"("error in"=w1765, "Filename (ini)"=w1768) -> ("error out"=w1764:errorcluster, "data"=w1767:T6)  [unwired: 8 in]
                n840 = Cluster To Array(cluster=w1767) -> (array=w1766:cluster{"Timing 0":dbl[]}[])
                n841 = for {
                  tunnel: w1766 -> [w1780] mode=indexing
                  tunnel: [w1769] -> w1763 mode=indexing
                  i -> [w1772]
                  n842 = To Double Precision Float(number=w1772) -> (double precision float=w1776:dbl)
                  n843 = Unbundle By Name(w1780) -> ("Timing 0"=w1779:dbl[])
                  n844 = Initialize Array(0.0 ("element"), 1 ("dimension size")) -> (w1773:dbl[])
                  n845 = Initialize Array(w1776, 1 ("dimension size")) -> (w1777:dbl[])
                  n846 = for {
                    tunnel: w1779 -> [w1782] mode=indexing
                    shift-right: [w1784] -> w1770
                    shift-left: w1777 -> [w1783]
                    shift-right: [w1786] -> w1771
                    shift-left: w1773 -> [w1785]
                    tunnel: w1772 -> [w1781]
                    i -> [w1791]
                    n847 = Quotient & Remainder(x=w1791, y=2) -> (x-y*floor(x/y)=w1789:i32)  [unwired: 1 out]
                    n848 = Equal To 0?(x=w1789) -> (x = 0?=w1788:bool)
                    n849 = Equal To 0?(x=w1782) -> (x = 0?=w1787:bool)
                    n850 = case shown="True" w1788 {
                      tunnel: w1787 -> [_ w1808]
                      tunnel: [w1792 w1807] -> w1786
                      tunnel: w1785 -> [w1794 w1806]
                      tunnel: [w1799 w1805] -> w1784
                      tunnel: w1783 -> [w1800 w1804]
                      tunnel: w1782 -> [w1795 w1803]
                      tunnel: w1781 -> [w1801 w1802]
                      frame False {
                        n851 = Array Size(array=w1794) -> (size(s)=w1798:i32)
                        n852 = Decrement(x=w1798) -> (x-1=w1797:i32)
                        n853 = Index Array(array=w1794, index=w1797) -> (element=w1796:dbl)
                        n854 = Build Array (concatenate)(w1800, w1801) -> (w1799:dbl[])
                        n855 = Add(x=w1795, y=w1796) -> (x+y=w1793:dbl)
                        n856 = Build Array (concatenate)(w1794, w1793) -> (w1792:dbl[])
                      }
                      frame True {
                        n857 = case shown="False" w1808 {
                          tunnel: [w1819 w1824] -> w1807
                          tunnel: w1806 -> [w1813 w1824]
                          tunnel: [w1815 w1823] -> w1805
                          tunnel: w1804 -> [w1822 w1823]
                          tunnel: w1803 -> [w1820 _]
                          tunnel: w1802 -> [w1816 _]
                          frame False {
                            n858 = Array Size(array=w1813) -> (size(s)=w1821:i32)
                            n859 = Add(x=0.5, y=w1816) -> (x+y=w1817:dbl)
                            n860 = Decrement(x=w1821) -> (x-1=w1814:i32)
                            n861 = Index Array(array=w1813, index=w1814) -> (element=w1811:dbl)
                            n862 = Add(x=w1820, y=w1811) -> (x+y=w1810:dbl)
                            n863 = Decrement(x=w1811) -> (x-1=w1812:dbl)
                            n864 = Build Array (concatenate)(w1822, w1816, w1817, w1817, w1816) -> (w1815:dbl[])
                            n865 = Decrement(x=w1810) -> (x-1=w1809:dbl)
                            n866 = Build Array (concatenate)(w1813, w1812, w1811, w1809, w1810) -> (w1819:dbl[])
                          }
                          frame True {
                          }
                        }
                      }
                    }
                  }
                  n867 = Bundle(w1771, w1770) -> (w1769:cluster{dbl[], dbl[]})  [unwired: 1 in]
                }
                "Pulses chart 2" <- w1763
              }
            }
          }
        }
      }
      event "Process_update": Mouse Down; "Process_show": Value Change {
        n868 = event-data() -> ()  [unwired: 1 in, 4 out]
        n869 = flat-sequence {
          tunnel: w1832 -> [w1839]
          tunnel: [w1838] -> w1834
          tunnel: "Config_Ver_2\\process\\processes\\" -> [w1835]
          tunnel: [w1835] -> w1828
          tunnel: "Config_Files\\" ("string") -> [w1836]
          tunnel: w1834 -> [w1847]
          tunnel: "Process_show" -> [w1846]
          tunnel: [w1847] -> w1830
          tunnel: [w1845] -> w1829
          tunnel: w1828 -> [w1845]
          tunnel: [w1844] -> w1827
          tunnel: w1830 -> [w1855]
          tunnel: w1829 -> [w1852]
          tunnel: w1827 -> [w1851]
          tunnel: [w1854] -> w1825
          frame #0 {
            # "Open the processes to the show the files"
            n870 = Concatenate Strings(w1836, w1835) -> (w1837:string)
            n871 = String To Path(string=w1837) -> (path=w1842:path)
            n872 = call <vilib>:"Application Directory.vi"() -> ("Application Directory"=w1843:path)
            n873 = Build Path(base path=w1843, name or relative path=w1842) -> (appended path=w1841:path)
            n874 = call <userlib>:"List Directory__ogtk.vi"("error in (no error)"=w1839, "directory path"=w1841) -> ("error out"=w1838:errorcluster, "file names"=w1840:string[])  [unwired: 2 in, 2 out]
            n875 = property on="Process_show" class="Ring (strict)"("Strings []"=w1840) -> ()  [unwired: 2 in, 2 out]
          }
          frame #1 {
            n876 = property on="Process_show" class="Ring (strict)"() -> ("Strings []"=w1848:string[])  [unwired: 2 in, 2 out]
            n877 = Index Array(array=w1848, index=w1846) -> (element=w1844:string)
            n878 = local write "Process name"(w1844) -> ()
          }
          frame #2 {
            n879 = String Length(string=w1851) -> (length=w1853:i32)
            n880 = Concatenate Strings(w1852, w1851) -> (w1849:string)
            n881 = Greater Than 0?(x=w1853) -> (x > 0?=w1850:bool)
            n882 = case shown="False" w1850 {
              tunnel: w1849 -> [_ w1862]
              tunnel: w1855 -> [w1856 w1859]
              tunnel: [w1856 w1858] -> w1854
              frame False {
              }
              frame True {
                n883 = call "Get_Pulse_Seq_DAQ.vi"("error in"=w1859, "Filename (ini)"=w1862) -> ("error out"=w1858:errorcluster, "data"=w1861:T6)  [unwired: 8 in]
                n884 = Cluster To Array(cluster=w1861) -> (array=w1860:cluster{"Timing 0":dbl[]}[])
                n885 = for {
                  tunnel: w1860 -> [w1874] mode=indexing
                  tunnel: [w1863] -> w1857 mode=indexing
                  i -> [w1866]
                  n886 = To Double Precision Float(number=w1866) -> (double precision float=w1870:dbl)
                  n887 = Unbundle By Name(w1874) -> ("Timing 0"=w1873:dbl[])
                  n888 = Initialize Array(0.0 ("element"), 1 ("dimension size")) -> (w1867:dbl[])
                  n889 = Initialize Array(w1870, 1 ("dimension size")) -> (w1871:dbl[])
                  n890 = for {
                    tunnel: w1873 -> [w1876] mode=indexing
                    shift-right: [w1878] -> w1864
                    shift-left: w1871 -> [w1877]
                    shift-right: [w1880] -> w1865
                    shift-left: w1867 -> [w1879]
                    tunnel: w1866 -> [w1875]
                    i -> [w1885]
                    n891 = Quotient & Remainder(x=w1885, y=2) -> (x-y*floor(x/y)=w1883:i32)  [unwired: 1 out]
                    n892 = Equal To 0?(x=w1883) -> (x = 0?=w1882:bool)
                    n893 = Equal To 0?(x=w1876) -> (x = 0?=w1881:bool)
                    n894 = case shown="False" w1882 {
                      tunnel: w1881 -> [_ w1902]
                      tunnel: [w1886 w1901] -> w1880
                      tunnel: w1879 -> [w1888 w1900]
                      tunnel: [w1893 w1899] -> w1878
                      tunnel: w1877 -> [w1894 w1898]
                      tunnel: w1876 -> [w1889 w1897]
                      tunnel: w1875 -> [w1895 w1896]
                      frame False {
                        n895 = Array Size(array=w1888) -> (size(s)=w1892:i32)
                        n896 = Decrement(x=w1892) -> (x-1=w1891:i32)
                        n897 = Index Array(array=w1888, index=w1891) -> (element=w1890:dbl)
                        n898 = Build Array (concatenate)(w1894, w1895) -> (w1893:dbl[])
                        n899 = Add(x=w1889, y=w1890) -> (x+y=w1887:dbl)
                        n900 = Build Array (concatenate)(w1888, w1887) -> (w1886:dbl[])
                      }
                      frame True {
                        n901 = case shown="True" w1902 {
                          tunnel: [w1913 w1918] -> w1901
                          tunnel: w1900 -> [w1907 w1918]
                          tunnel: [w1909 w1917] -> w1899
                          tunnel: w1898 -> [w1916 w1917]
                          tunnel: w1897 -> [w1914 _]
                          tunnel: w1896 -> [w1910 _]
                          frame False {
                            n902 = Array Size(array=w1907) -> (size(s)=w1915:i32)
                            n903 = Add(x=0.5, y=w1910) -> (x+y=w1911:dbl)
                            n904 = Decrement(x=w1915) -> (x-1=w1908:i32)
                            n905 = Index Array(array=w1907, index=w1908) -> (element=w1905:dbl)
                            n906 = Add(x=w1914, y=w1905) -> (x+y=w1904:dbl)
                            n907 = Decrement(x=w1905) -> (x-1=w1906:dbl)
                            n908 = Build Array (concatenate)(w1916, w1910, w1911, w1911, w1910) -> (w1909:dbl[])
                            n909 = Decrement(x=w1904) -> (x-1=w1903:dbl)
                            n910 = Build Array (concatenate)(w1907, w1906, w1905, w1903, w1904) -> (w1913:dbl[])
                          }
                          frame True {
                          }
                        }
                      }
                    }
                  }
                  n911 = Bundle(w1865, w1864) -> (w1863:cluster{dbl[], dbl[]})  [unwired: 1 in]
                }
                "Pulses chart 3" <- w1857
              }
            }
          }
        }
      }
      event "Choose init states": Mouse Down {
        n912 = event-data() -> ()  [unwired: 1 in, 8 out]
        n913 = local read "Initial_state_name"() -> (w1928:string)
        n914 = local read "Config folder"() -> (w1919:string)
        n915 = String Length(string=w1928) -> (length=w1929:i32)
        n916 = Greater Than 0?(x=w1929) -> (x > 0?=w1920:bool)
        n917 = Concatenate Strings(w1919, "\\state_library\\", w1928) -> (w1922:string)
        n918 = Concatenate Strings(w1919, "\\process\\init_states_sets\\") -> (w1926:string)
        n919 = case shown="True" w1920 {
          tunnel: w1930 -> [w1931 w1941]
          tunnel: w1928 -> [_ w1940]
          tunnel: w1926 -> [_ w1939]
          tunnel: [w1931 w1938] -> w1924
          tunnel: w1922 -> [_ w1937]
          frame False {
          }
          frame True {
            n920 = call "Get_Pulse_Seq_DAQ.vi"("error in"=w1941, "Filename (ini)"=w1937) -> ("error out"=w1935:errorcluster, "data"=w1936:T6)  [unwired: 8 in]
            n921 = local read "Sampling data"() -> (w1934:T2)
            n922 = Concatenate Strings(w1939, w1940) -> (w1932:string)
            n923 = call "Set_Pulse_Seq_DAQ.vi"("Time Unit"=T12 {"Time Unit"=enum."MicroSecond"}, "error in"=w1935, "Sampling data"=w1934, "Sequence"=w1936, "Filename (ini)"=w1932) -> ("error out"=w1938:errorcluster)  [unwired: 6 in]
          }
        }
        n924 = call "Read_filename.vi"("error in"=w1924, "Filename (ini)"=w1926) -> ("error out"=w1925:errorcluster, "Strings []"=w1927:string[])  [unwired: 8 in]
        n925 = local write "State_List"(w1927) -> ()
      }
      event "Choose the process": Mouse Down {
        n926 = event-data() -> ()  [unwired: 1 in, 8 out]
        n927 = local read "Process name"() -> (w1947:string)
        n928 = local read "Config folder"() -> (w1942:string)
        n929 = String Length(string=w1947) -> (length=w1948:i32)
        n930 = Greater Than 0?(x=w1948) -> (x > 0?=w1944:bool)
        n931 = Concatenate Strings(w1942, "\\process\\processes\\") -> (w1946:string)
        n932 = case shown="True" w1944 {
          tunnel: w1949 -> [w1950 w1957]
          tunnel: w1947 -> [_ w1956]
          tunnel: w1946 -> [_ w1955]
          tunnel: [w1950 w1952] -> w1943
          frame False {
          }
          frame True {
            n933 = Concatenate Strings(w1955, w1956) -> (w1954:string)
            n934 = call "Get_Pulse_Seq_DAQ.vi"("error in"=w1957, "Filename (ini)"=w1954) -> ("error out"=w1952:errorcluster, "data"=w1953:T6)  [unwired: 8 in]
            n935 = call "Squence_to_Array_SubVI.vi"("Sequence"=w1953) -> ("Array"=w1951:cluster{"Timing 0":dbl[]}[])  [unwired: 10 in]
            n936 = local write "Process Array"(w1951) -> ()
            "The Choosen Process" <- w1956
          }
        }
      }
      event "Delete init states": Mouse Down {
        # "Check the name if it's in the State_list, if yes, the name will be deleted, otherwise, return"
        n937 = event-data() -> ()  [unwired: 1 in, 8 out]
        n938 = local read "Initial_state_name"() -> (w1963:string)
        n939 = local read "Config folder"() -> (w1958:string)
        n940 = local read "State_List"() -> (w1965:string[])
        n941 = Concatenate Strings(w1958, "\\process\\init_states_sets\\") -> (w1966:string)
        n942 = for {
          tunnel: w1965 -> [w1978] mode=indexing
          shift-right: [w1974] -> w1962
          shift-left: FALSE -> [w1975]
          tunnel: w1963 -> [w1977]
          n943 = Equal?(x=w1977, y=w1978) -> (x = y?=w1976:bool)
          n944 = Or(x=w1975, y=w1976) -> (x .or. y?=w1974:bool)
        }
        n945 = Concatenate Strings(w1966, w1963) -> (w1959:string)
        n946 = case shown="True" w1962 {
          tunnel: w1961 -> [w1970 w1971]
          tunnel: [w1970 w1973] -> w1960
          tunnel: w1959 -> [_ w1972]
          frame False {
          }
          frame True {
            n947 = call "Delete_file.vi"("error in"=w1971, "Filename (ini)"=w1972) -> ("error out"=w1973:errorcluster)  [unwired: 9 in]
          }
        }
        n948 = call "Read_filename.vi"("error in"=w1960, "Filename (ini)"=w1966) -> ("error out"=w1968:errorcluster, "Strings []"=w1969:string[])  [unwired: 8 in]
        n949 = local write "State_List"(w1969) -> ()
      }
      event "Clear All states": Mouse Down {
        n950 = event-data() -> ()  [unwired: 1 in, 8 out]
        n951 = local read "Config folder"() -> (w1986:string)
        n952 = local read "State_List"() -> (w1985:string[])
        n953 = Concatenate Strings(w1986, "\\process\\init_states_sets\\") -> (w1980:string)
        n954 = Array Size(array=w1985) -> (size(s)=w1984:i32)
        n955 = Greater Than 0?(x=w1984) -> (x > 0?=w1983:bool)
        n956 = flat-sequence {
          tunnel: w1980 -> [w1992]
          tunnel: w1985 -> [w1991]
          tunnel: w1983 -> [w1990]
          tunnel: w1982 -> [w1989]
          tunnel: [w1988] -> w1981
          tunnel: w1981 -> [w2005]
          tunnel: w1980 -> [w2004]
          tunnel: [w2003] -> w1979
          frame #0 {
            n957 = case shown="False" w1990 {
              tunnel: w1992 -> [_ w1997]
              tunnel: w1991 -> [_ w1996]
              tunnel: w1989 -> [w1993 w1995]
              tunnel: [w1993 w1994] -> w1988
              frame False {
              }
              frame True {
                n958 = for {
                  tunnel: w1996 -> [w2001] mode=indexing
                  tunnel: w1997 -> [w2002]
                  shift-right: [w1998] -> w1994
                  shift-left: w1995 -> [w1999]
                  n959 = Concatenate Strings(w2002, w2001) -> (w2000:string)
                  n960 = call "Delete_file.vi"("error in"=w1999, "Filename (ini)"=w2000) -> ("error out"=w1998:errorcluster)  [unwired: 9 in]
                }
              }
            }
          }
          frame #1 {
            n961 = call "Read_filename.vi"("error in"=w2005, "Filename (ini)"=w2004) -> ("error out"=w2003:errorcluster, "Strings []"=w2006:string[])  [unwired: 8 in]
            n962 = local write "State_List"(w2006) -> ()
          }
        }
      }
      event "Show init state": Mouse Down {
        n963 = event-data() -> ()  [unwired: 1 in, 8 out]
        n964 = local read "Config folder"() -> (w2007:string)
        n965 = Concatenate Strings(w2007, "\\process\\init_states_sets\\") -> (w2011:string)
        n966 = call "Read_filename.vi"("error in"=w2010, "Filename (ini)"=w2011) -> ("error out"=w2009:errorcluster, "Strings []"=w2008:string[])  [unwired: 8 in]
        n967 = local write "State_List"(w2008) -> ()
      }
      event "Reset sequence": Mouse Down {
        n968 = event-data() -> ()  [unwired: 1 in, 8 out]
        n969 = Wait (ms)(milliseconds to wait=u32 150) -> ()  [unwired: 1 out]
      }
    }
  }
